vi "UI Main - SuNLaMP v1.3.0.vi"() -> ()   [LabVIEW 2017]
uses:
  e1ad3939-0f1a-413b-8e12-73ea7a7ed0d6.vi
  13f53db5-d547-40ce-b72e-27caf69f0b89.vi
  76f48c83-6457-427b-80e1-e30a4e2751fa.vi
  Globals/Global - All UI Loop Stop.vi
  support/Match 1D Array Elements/Match 1D Array Elements - string.vi
  support/Delete Elements From Array/Delete Elements From Array - double.vi
  Globals/Global - Configuration Options.vi
  Globals/Global - UI Stream and Variable Connections.vi
  support/User Event - Stop/User Event - Stop.lvlib
  support/Message Queue/Message Queue.lvlib
panel:
  in  "Temp To Monitor":string="Recup Cold Outlet Temperature [F]\nRecup Hot Inlet Temperature [F]\nPump Outlet Temperature [F]\nPump Inlet Temperature [F]\nCooler Outlet Temperature [F]\nCooler Inlet Temperature [F]\nWater Inlet Temperature [F]\nWater Outlet Temperature [F]\nRecup Hot Outlet Temperature [F]\nRecup Cold Inlet Temperature [F]\nHeater Inlet Temperature [F]"
  in  "Temp Alert Limit":dbl=140.0 format="%#_13g"
  in  "Alarm":bool
  in  "Temp Alert":bool
  out "time":timestamp format="%<%Y-%m-%d %H:%M:%S%2u>T"
  in  "clear?":bool
  in  "pump map":path=path "C:/LabView/7.5 hp Magnepump Curves.txt"
  in  "Refresh Map?":bool
  out "Map":cluster{dbl[], dbl[]}[](graph)=[{[15.211267605633802], [164.25819822966048]}, {[15.211267605633802, 15.211267605633802, 15.211267605633802, 15.211267605633802, 15.211267605633802, 15.211267605633802, 15.211267605633802, 15.211267605633802, 15.211267605633802, 15.211267605633802, 15.211267605633802, 15.211267605633802, 15.211267605633802, 15.211267605633802, 15.211267605633802, 15.211267605633802, 15.211267605633802, 15.211267605633802, 15.211267605633802, 15.211267605633802, 15.211267605633802, 15.211267605633802, 15.211267605633802, 15.211267605633802, 15.211267605633802, 15.211267605633802, 15.211267605633802, 15.211267605633802, 15.211267605633802, 15.211267605633802, 15.211267605633802, 15.211267605633802, 15.211267605633802, 15.211267605633802, 15.211267605633802, 15.211267605633802, 15.211267605633802, 15.211267605633802, 15.211267605633802, 15.211267605633802, 15.211267605633802, 15.211267605633802, 15.211267605633802, 15.211267605633802, 15.211267605633802, 15.211267605633802, 15.211267605633802, 15.211267605633802, 15.211267605633802, 15.211267605633802, 15.211267605633802, 15.211267605633802, 15.211267605633802, 15.211267605633802, 15.211267605633802, 15.211267605633802, 15.211267605633802, 15.211267605633802, 15.211267605633802, 15.211267605633802, 15.211267605633802, 15.211267605633802, 15.211267605633802, 15.211267605633802, 15.211267605633802, 15.211267605633802, 15.211267605633802, 15.211267605633802, 15.211267605633802, 15.211267605633802, 15.211267605633802, 15.211267605633802, 15.211267605633802], [164.25819822966048, 164.25819822966048, 164.25819822966048, 164.25819822966048, 164.25819822966048, 164.25819822966048, 164.25819822966048, 164.25819822966048, 164.25819822966048, 164.25819822966048, 164.25819822966048, 164.25819822966048, 164.25819822966048, 164.25819822966048, 164.25819822966048, 164.25819822966048, 164.25819822966048, 164.25819822966048, 164.25819822966048, 164.25819822966048, 164.25819822966048, 164.25819822966048, 164.25819822966048, 164.25819822966048, 164.25819822966048, 164.25819822966048, 164.25819822966048, 164.25819822966048, 164.25819822966048, 164.25819822966048, 164.25819822966048, 164.25819822966048, 164.25819822966048, 164.25819822966048, 164.25819822966048, 164.25819822966048, 164.25819822966048, 164.25819822966048, 164.25819822966048, 164.25819822966048, 164.25819822966048, 164.25819822966048, 164.25819822966048, 164.25819822966048, 164.25819822966048, 164.25819822966048, 164.25819822966048, 164.25819822966048, 164.25819822966048, 164.25819822966048, 164.25819822966048, 164.25819822966048, 164.25819822966048, 164.25819822966048, 164.25819822966048, 164.25819822966048, 164.25819822966048, 164.25819822966048, 164.25819822966048, 164.25819822966048, 164.25819822966048, 164.25819822966048, 164.25819822966048, 164.25819822966048, 164.25819822966048, 164.25819822966048, 164.25819822966048, 164.25819822966048, 164.25819822966048, 164.25819822966048, 164.25819822966048, 164.25819822966048, 164.25819822966048]}, {[0.0, 0.5050505050505051, 1.0101010101010102, 1.5151515151515151, 2.0202020202020203, 2.525252525252525, 3.0303030303030303, 3.535353535353535, 4.040404040404041, 4.545454545454546, 5.05050505050505, 5.555555555555555, 6.0606060606060606, 6.565656565656567, 7.07070707070707, 7.575757575757576, 8.080808080808081, 8.585858585858585, 9.090909090909092, 9.595959595959595, 10.1010101010101, 10.606060606060606, 11.11111111111111, 11.616161616161616, 12.121212121212121, 12.626262626262626, 13.131313131313133, 13.636363636363635, 14.14141414141414, 14.646464646464647, 15.151515151515152, 15.656565656565657, 16.161616161616163, 16.666666666666664, 17.17171717171717, 17.67676767676768, 18.181818181818183, 18.68686868686869, 19.19191919191919, 19.696969696969695, 20.2020202020202, 20.707070707070706, 21.21212121212121, 21.71717171717172, 22.22222222222222, 22.727272727272727, 23.232323232323232, 23.737373737373737, 24.242424242424242, 24.747474747474747, 25.252525252525253, 25.757575757575758, 26.262626262626267, 26.767676767676768, 27.27272727272727, 27.77777777777778, 28.28282828282828, 28.78787878787879, 29.292929292929294, 29.797979797979796, 30.303030303030305, 30.808080808080806, 31.313131313131315, 31.818181818181817, 32.323232323232325, 32.82828282828283, 33.33333333333333, 33.83838383838384, 34.34343434343434, 34.84848484848485, 35.35353535353536, 35.858585858585855, 36.36363636363637, 36.868686868686865, 37.37373737373738, 37.878787878787875, 38.38383838383838, 38.88888888888889, 39.39393939393939, 39.8989898989899, 40.4040404040404, 40.909090909090914, 41.41414141414141, 41.91919191919192, 42.42424242424242, 42.92929292929293, 43.43434343434344, 43.93939393939394, 44.44444444444444, 44.94949494949495, 45.45454545454545, 45.95959595959596, 46.464646464646464, 46.96969696969697, 47.474747474747474, 47.97979797979798, 48.484848484848484, 48.98989898989899, 49.494949494949495, 50.0], [320.0, 319.9999997193249, 319.99999455484533, 319.99996914478146, 319.9998943628826, 319.9997255914889, 319.99940140243217, 319.99884246717903, 319.99795061825614, 319.9966080194432, 319.9946764186028, 319.99199646578484, 319.9883870844086, 319.98364488659047, 319.977543625857, 319.96983368198966, 319.960241573831, 319.9484694966772, 319.9341948814863, 319.9170699735952, 319.8967214290018, 319.87274992655915, 319.8447297946612, 319.8122086511911, 319.7747070556596, 319.7317181725931, 319.68270744533976, 319.62711227955526, 319.5643417357107, 319.4937762300317, 319.41476724333677, 319.32663703729554, 319.22867837767024, 319.1201542641441, 319.0002976663747, 318.86831126594063, 318.72336720387625, 318.56460683351537, 318.3911404783842, 318.20204719490437, 317.99637453968427, 317.7731383411927, 317.5313224756226, 317.269878646766, 316.987726169734, 316.6837517583631, 316.35680931616446, 316.00571973067593, 315.62927067108876, 315.226216389027, 314.7952775223654, 314.33514090197644, 313.8444593613058, 313.32185154867767, 312.76590174224026, 312.1751596674631, 311.5481403171046, 310.8833237735713, 310.17915503359444, 309.43404383515303, 308.64636448657575, 307.8144556977579, 306.9366204134314, 306.0111256484296, 305.03620232489067, 304.0100451113468, 302.9308122636464, 301.7966254676617, 300.6055696837347, 299.35569299281417, 298.0450064442441, 296.67148390515854, 295.23306191144485, 293.72763952023706, 292.15307816390055, 290.5072015054755, 288.7877952955416, 286.99260723047416, 285.1193468120571, 283.1656852084245, 281.1292551162997, 279.0076506245035, 276.7984270787053, 274.49910094738806, 272.1071496890043, 269.6200116202959, 267.0350857857544, 264.3497318281997, 261.561269860452, 258.6669803380781, 255.6641039331887, 252.54984140926717, 249.32135349701005, 245.97576077115912, 242.51014352830754, 238.92154166566087, 235.20695456073582, 231.36334095197986, 227.38761882029425, 223.27666527144538]}, {[0.0, 0.4951475539710834, 0.9902951079421668, 1.4854426619132501, 1.9805902158843336, 2.475737769855417, 2.9708853238265003, 3.4660328777975833, 3.961180431768667, 4.456327985739751, 4.951475539710834, 5.446623093681917, 5.941770647653001, 6.436918201624085, 6.932065755595167, 7.427213309566251, 7.922360863537334, 8.417508417508417, 8.912655971479502, 9.407803525450584, 9.902951079421667, 10.39809863339275, 10.893246187363834, 11.388393741334918, 11.883541295306001, 12.378688849277085, 12.87383640324817, 13.36898395721925, 13.864131511190333, 14.359279065161418, 14.854426619132502, 15.349574173103585, 15.844721727074669, 16.339869281045747, 16.835016835016834, 17.33016438898792, 17.825311942959004, 18.320459496930088, 18.815607050901168, 19.31075460487225, 19.805902158843335, 20.301049712814418, 20.7961972667855, 21.29134482075659, 21.78649237472767, 22.281639928698752, 22.776787482669835, 23.27193503664092, 23.767082590612002, 24.262230144583086, 24.75737769855417, 25.252525252525253, 25.74767280649634, 26.24282036046742, 26.7379679144385, 27.233115468409586, 27.728263022380666, 28.223410576351753, 28.718558130322837, 29.213705684293917, 29.708853238265004, 30.204000792236084, 30.69914834620717, 31.19429590017825, 31.689443454149337, 32.18459100812042, 32.679738562091494, 33.17488611606259, 33.67003367003367, 34.165181224004755, 34.66032877797584, 35.155476331946915, 35.65062388591801, 36.14577143988908, 36.640918993860176, 37.13606654783125, 37.631214101802335, 38.12636165577342, 38.6215092097445, 39.11665676371559, 39.61180431768667, 40.106951871657756, 40.602099425628836, 41.097246979599916, 41.592394533571, 42.08754208754208, 42.58268964151318, 43.07783719548425, 43.57298474945534, 44.06813230342642, 44.563279857397504, 45.058427411368584, 45.55357496533967, 46.04872251931075, 46.54387007328184, 47.03901762725292, 47.534165181224004, 48.029312735195084, 48.52446028916617, 49.01960784313725], [307.5740099961553, 307.57400972637913, 307.5740047624426, 307.5739803390825, 307.57390846105596, 307.57374624326116, 307.5734346428606, 307.5728974117445, 307.5720401944023, 307.5707497303376, 307.56889313591194, 307.5663172489281, 307.5628480242297, 307.55828997173245, 307.5524256303892, 307.5450150730389, 307.5357954381305, 307.52448048507995, 307.51076017059427, 307.4943002437478, 307.47474185794096, 307.4517011981537, 307.4247691221272, 307.3935108142936, 307.3574654514221, 307.3161458790783, 307.26903829809663, 307.2156019603568, 307.1552688732321, 307.0874435121412, 307.01150254069273, 306.9267945379619, 306.83263973247807, 306.72832974254527, 306.6131273225439, 306.4862661148987, 306.3469504074166, 306.19435489572794, 306.02762445058073, 305.84587388975814, 305.64818775440625, 305.4336200895739, 305.20119422877985, 304.9499025824356, 304.6787064299635, 304.38653571545854, 304.0722888467555, 303.73483249776615, 303.3730014139646, 302.98559822090255, 302.5713932356453, 302.1291242810231, 301.6574965026007, 301.1551821882715, 300.6208205903885, 300.053017750349, 299.45034632555223, 298.81134541865754, 298.13452040906805, 297.41834278657535, 296.661249987097, 295.86164523044783, 295.01789736008396, 294.1283406847651, 293.19127482207864, 292.20496454377815, 291.16763962288195, 290.07749468248915, 288.9326890462656, 287.7313465905557, 286.4715555980816, 285.1513686131858, 283.7688022985821, 282.32183729357655, 280.8084180737221, 279.22645281187573, 277.57381324062055, 275.8483345160267, 274.0478150827154, 272.1700165402004, 270.21266351047643, 268.17344350682765, 266.0500068038305, 263.8399663085237, 261.5408974327223, 259.1503379664512, 256.66578795247443, 254.08470956189896, 251.40452697083043, 248.6226262380604, 245.7363551837646, 242.7430232691918, 239.63990147732605, 236.42422219450125, 233.09317909295225, 229.64392701428378, 226.07358185384064, 222.37922044596294, 218.5578804501098, 214.60656023783676]}, {[0.0, 0.4621377170396778, 0.9242754340793556, 1.3864131511190334, 1.8485508681587113, 2.3106885851983887, 2.772826302238067, 3.2349640192777445, 3.6971017363174226, 4.159239453357101, 4.621377170396777, 5.083514887436456, 5.545652604476134, 6.007790321515812, 6.469928038555489, 6.9320657555951675, 7.394203472634845, 7.856341189674522, 8.318478906714201, 8.780616623753877, 9.242754340793555, 9.704892057833234, 10.167029774872912, 10.62916749191259, 11.091305208952267, 11.553442925991945, 12.015580643031624, 12.4777183600713, 12.939856077110978, 13.401993794150657, 13.864131511190335, 14.326269228230013, 14.78840694526969, 15.250544662309366, 15.712682379349044, 16.174820096388725, 16.636957813428403, 17.09909553046808, 17.561233247507754, 18.023370964547432, 18.48550868158711, 18.947646398626787, 19.40978411566647, 19.87192183270615, 20.334059549745824, 20.7961972667855, 21.25833498382518, 21.720472700864857, 22.182610417904534, 22.644748134944212, 23.10688585198389, 23.569023569023567, 24.03116128606325, 24.493299003102923, 24.9554367201426, 25.41757443718228, 25.879712154221956, 26.341849871261637, 26.803987588301315, 27.26612530534099, 27.72826302238067, 28.190400739420344, 28.652538456460025, 29.1146761734997, 29.57681389053938, 30.038951607579058, 30.501089324618732, 30.963227041658417, 31.425364758698088, 31.887502475737772, 32.34964019277745, 32.811777909817124, 33.273915626856805, 33.73605334389648, 34.19819106093616, 34.660328777975835, 35.12246649501551, 35.5846042120552, 36.046741929094864, 36.50887964613455, 36.97101736317422, 37.43315508021391, 37.895292797253575, 38.357430514293256, 38.81956823133294, 39.28170594837261, 39.7438436654123, 40.20598138245197, 40.66811909949165, 41.13025681653132, 41.592394533571, 42.05453225061068, 42.51666996765036, 42.97880768469003, 43.440945401729714, 43.90308311876939, 44.36522083580907, 44.82735855284875, 45.289496269888424, 45.751633986928105], [267.93113759665084, 267.9311373616458, 267.93113303750556, 267.9311117620452, 267.93104914829763, 267.93090783857417, 267.930636400003, 267.9301684120085, 267.9294216804571, 267.9282975428718, 267.9266802428388, 267.92443635906625, 267.9214142788845, 267.91744370870913, 267.91233521580574, 267.9058797969583, 267.89784847054926, 267.8879918892252, 267.87603997082874, 267.8617015456647, 267.844664018473, 267.82459304372503, 267.80113221305305, 267.7739027537846, 267.74250323768325, 267.70650929910823, 267.6654733618975, 267.6189243743553, 267.5663675517933, 267.5072841261319, 267.4411311021146, 267.36734101973565, 267.28532172251425, 267.19445613128386, 267.0941020231938, 266.98359181564507, 266.86223235490513, 266.7293047091674, 266.5840639658392, 266.425739032856, 266.2535324438383, 266.0666201669177, 265.86415141707045, 265.64524847181053, 265.4090064901015, 265.154493334355, 264.8807493953959, 264.58678742027627, 264.27159234283135, 263.9341211168751, 263.5733025519399, 263.18803715146896, 262.7771969533766, 262.33962537289426, 261.87413704762736, 261.3795176847484, 260.8545239102588, 260.2978831202528, 259.7082933341215, 259.084423049639, 258.42491109987117, 257.72836651185673, 256.9933683670065, 256.2184656631731, 255.40217717834406, 254.5429913359134, 253.63936607148824, 252.68972870119052, 251.69247579141353, 250.64597302999516, 249.54855509877328, 248.3985255474863, 247.19415666898706, 245.93368937573777, 244.61533307755352, 243.23726556056727, 241.79763286738498, 240.29454917840545, 238.72609669427646, 237.09032551946345, 235.3852535469039, 233.60886634372542, 231.75911703800347, 229.83392620653618, 227.83118176361586, 225.74873885077528, 223.5844197274888, 221.33601366280976, 219.0012768279234, 216.5779321895993, 214.0636694045238, 211.45614471449596, 208.7529808424707, 205.95176688943218, 203.05005823208285, 200.04537642133164, 196.93520908156785, 193.7170098107055, 190.38819808098452, 186.94615914051556]}, {[0.0, 0.4291278801082723, 0.8582557602165446, 1.2873836403248167, 1.7165115204330892, 2.145639400541361, 2.5747672806496333, 3.0038951607579056, 3.4330230408661784, 3.8621509209744507, 4.291278801082722, 4.720406681190995, 5.149534561299267, 5.57866244140754, 6.007790321515811, 6.436918201624084, 6.866046081732357, 7.295173961840628, 7.724301841948901, 8.153429722057172, 8.582557602165444, 9.011685482273716, 9.44081336238199, 9.869941242490262, 10.299069122598533, 10.728197002706807, 11.15732488281508, 11.586452762923349, 12.015580643031623, 12.444708523139896, 12.873836403248168, 13.30296428335644, 13.732092163464714, 14.161220043572982, 14.590347923681255, 15.01947580378953, 15.448603683897803, 15.877731564006075, 16.306859444114345, 16.735987324222616, 17.16511520433089, 17.59424308443916, 18.023370964547432, 18.452498844655707, 18.88162672476398, 19.31075460487225, 19.739882484980523, 20.169010365088795, 20.598138245197067, 21.027266125305342, 21.456394005413614, 21.885521885521886, 22.31464976563016, 22.74377764573843, 23.172905525846698, 23.602033405954973, 24.031161286063245, 24.46028916617152, 24.889417046279792, 25.31854492638806, 25.747672806496336, 26.176800686604604, 26.60592856671288, 27.03505644682115, 27.464184326929427, 27.8933122070377, 28.322440087145964, 28.751567967254243, 29.18069584736251, 29.609823727470786, 30.03895160757906, 30.468079487687326, 30.897207367795605, 31.32633524790387, 31.75546312801215, 32.184591008120414, 32.61371888822869, 33.042846768336965, 33.47197464844523, 33.90110252855351, 34.33023040866178, 34.75935828877006, 35.18848616887832, 35.617614048986596, 36.046741929094864, 36.47586980920314, 36.904997689311415, 37.33412556941968, 37.76325344952796, 38.19238132963623, 38.6215092097445, 39.05063708985278, 39.479764969961046, 39.90889285006932, 40.33802073017759, 40.767148610285865, 41.19627649039413, 41.62540437050241, 42.054532250610684, 42.48366013071895], [231.02225639711222, 231.02225619448035, 231.02225246601247, 231.02223412135532, 231.02218013297093, 231.02205828938284, 231.02182424285974, 231.02142072259923, 231.02077685712882, 231.01980757523134, 231.01841306652943, 231.0164782891949, 231.01387251597697, 231.01044891210128, 231.00604414015905, 231.00047798819364, 230.9935530179736, 230.98505423101562, 230.97474875035746, 230.96238551641497, 230.9476949955201, 230.9303888999466, 230.9101599183978, 230.88668145606943, 230.8596073835126, 230.82857179361883, 230.79318876612592, 230.75305213911247, 230.70773528700545, 230.65679090467495, 230.59975079723145, 230.53612567518024, 230.4654049546169, 230.38705656217846, 230.30052674448854, 230.20523988185727, 230.10059830601514, 229.9859821216801, 229.86074903176953, 229.72423416608498, 229.57574991330958, 229.41458575616883, 229.24000810961687, 229.0512601619183, 228.8475617185059, 228.6281090485, 228.39207473378525, 228.13860752054438, 227.86683217315561, 227.5758493303668, 227.26473536366248, 226.93254223774625, 226.57829737306452, 226.2010035103017, 225.79963857678072, 225.37315555470659, 224.9204823511926, 224.44052167001388, 223.93215088503337, 223.39422191524994, 222.82556110141954, 222.22496908420302, 221.59122068379642, 220.92306478100133, 220.21922419969465, 219.47839559066006, 218.69924931674242, 217.88042933929185, 217.0205531058617, 216.11821143912852, 215.17196842700352, 214.18036131390403, 213.14190039315724, 212.05506890050862, 210.91832290870687, 209.7300912231422, 208.48877527851056, 207.19274903648227, 205.84035888435065, 204.4299235346394, 202.95973392564676, 201.42805312290614, 199.8331162215438, 198.17313024951335, 196.4462740716892, 194.65069829480115, 192.7845251731919, 190.8458485153819, 188.83273359142376, 186.74321704103207, 184.57530678247207, 182.32698192219297, 179.9961926651916, 177.58086022609206, 175.0788767409286, 172.4881051796176, 169.806379259107, 167.03150335718996, 164.16125242697137, 161.19337191197516]}, {[0.0, 0.3961180431768667, 0.7922360863537334, 1.1883541295306002, 1.5844721727074669, 1.9805902158843334, 2.3767082590612003, 2.772826302238067, 3.1689443454149337, 3.5650623885918007, 3.9611804317686667, 4.357298474945534, 4.753416518122401, 5.149534561299268, 5.545652604476134, 5.941770647653001, 6.3378886908298675, 6.734006734006733, 7.130124777183601, 7.5262428203604665, 7.9223608635373335, 8.3184789067142, 8.714596949891067, 9.110714993067933, 9.506833036244801, 9.902951079421667, 10.299069122598535, 10.6951871657754, 11.091305208952267, 11.487423252129135, 11.883541295306001, 12.279659338482869, 12.675777381659735, 13.0718954248366, 13.468013468013465, 13.864131511190335, 14.260249554367203, 14.656367597544069, 15.052485640720933, 15.448603683897801, 15.844721727074667, 16.240839770251533, 16.6369578134284, 17.03307585660527, 17.429193899782135, 17.825311942959, 18.221429986135867, 18.617548029312733, 19.013666072489602, 19.40978411566647, 19.805902158843335, 20.2020202020202, 20.59813824519707, 20.994256288373936, 21.3903743315508, 21.78649237472767, 22.182610417904534, 22.578728461081404, 22.97484650425827, 23.370964547435133, 23.767082590612002, 24.16320063378887, 24.559318676965738, 24.9554367201426, 25.35155476331947, 25.747672806496336, 26.1437908496732, 26.53990889285007, 26.93602693602693, 27.332144979203804, 27.72826302238067, 28.124381065557532, 28.520499108734406, 28.916617151911264, 29.312735195088138, 29.708853238265, 30.104971281441866, 30.50108932461874, 30.897207367795602, 31.29332541097247, 31.689443454149334, 32.0855614973262, 32.481679540503066, 32.877797583679936, 33.2739156268568, 33.67003367003367, 34.06615171321054, 34.4622697563874, 34.85838779956427, 35.25450584274113, 35.650623885918, 36.04674192909487, 36.442859972271734, 36.8389780154486, 37.235096058625466, 37.631214101802335, 38.027332144979205, 38.42345018815607, 38.81956823133294, 39.21568627450981], [196.8473663975394, 196.84736622488265, 196.84736304796328, 196.8473474170128, 196.8473014150758, 196.84719759568713, 196.84699817143078, 196.8466543435165, 196.84610572441744, 196.84527982741605, 196.84409160698365, 196.842443039314, 196.840222735507, 196.83730558190877, 196.83355240344912, 196.82880964674487, 196.82290908040352, 196.81566751045116, 196.80688650918032, 196.79635215599856, 196.78383478908222, 196.76908876681838, 196.75185223816143, 196.7318469211479, 196.70877788891013, 196.68233336261014, 196.65218451078184, 196.61798525462837, 196.57937207886854, 196.53596384777035, 196.48736162604337, 196.4331485042956, 196.37288942878598, 196.30613103522896, 196.2324014864281, 196.15121031353516, 196.06204826074662, 195.9643871332659, 195.85767964837166, 195.7413592894452, 195.61484016282, 195.4775168573273, 195.32876430641912, 195.16793765275878, 194.99437211517662, 194.80738285789346, 194.60626486192353, 194.39029279857036, 194.15872090493733, 193.9107828613776, 193.645691670813, 193.36263953985477, 193.06079776166445, 192.73931660049374, 192.39732517784867, 192.03393136022336, 191.64822164835346, 191.23926106794082, 190.80609306180358, 190.34773938340822, 189.86319999174208, 189.3514529474866, 188.81145431045374, 188.24213803824964, 187.64241588613035, 187.01117730801803, 186.34728935864445, 185.64959659679306, 184.91692098960996, 184.14806181795564, 183.34179558277222, 182.49687591243892, 181.61203347109256, 180.685975867889, 179.7173875671822, 178.70492979960045, 177.64724047399716, 176.54293409025706, 175.39060165293782, 174.18881058572825, 172.93610464670493, 171.6310038443697, 170.27200435445152, 168.85757843745515, 167.38617435694226, 165.85621629852878, 164.26610428958364, 162.61421411961535, 160.89889726133148, 159.11848079235867, 157.27126731760933, 155.35553489228275, 153.36953694548868, 151.3115022044808, 149.17963461948943, 146.97211328914162, 144.687092386458, 142.3227010854163, 139.87704348807029, 137.34819855221554]}, {[0.0, 0.3631082062454612, 0.7262164124909224, 1.0893246187363834, 1.4524328249818448, 1.8155410312273057, 2.178649237472767, 2.541757443718228, 2.9048656499636896, 3.2679738562091507, 3.6310820624546114, 3.9941902687000725, 4.357298474945534, 4.720406681190996, 5.083514887436456, 5.446623093681917, 5.809731299927379, 6.1728395061728385, 6.535947712418301, 6.899055918663761, 7.262164124909223, 7.625272331154684, 7.988380537400145, 8.351488743645605, 8.714596949891067, 9.07770515613653, 9.440813362381991, 9.80392156862745, 10.167029774872912, 10.530137981118374, 10.893246187363834, 11.256354393609296, 11.619462599854758, 11.982570806100217, 12.345679012345677, 12.70878721859114, 13.071895424836603, 13.435003631082063, 13.798111837327522, 14.161220043572984, 14.524328249818446, 14.887436456063906, 15.250544662309368, 15.613652868554832, 15.97676107480029, 16.33986928104575, 16.70297748729121, 17.066085693536674, 17.429193899782135, 17.792302106027595, 18.15541031227306, 18.51851851851852, 18.881626724763983, 19.24473493100944, 19.6078431372549, 19.970951343500364, 20.334059549745824, 20.697167755991288, 21.060275962236748, 21.423384168482205, 21.78649237472767, 22.14960058097313, 22.512708787218592, 22.875816993464053, 23.238925199709517, 23.602033405954977, 23.965141612200433, 24.328249818445897, 24.691358024691354, 25.05446623093682, 25.41757443718228, 25.78068264342774, 26.143790849673206, 26.506899055918662, 26.870007262164126, 27.233115468409583, 27.596223674655043, 27.95933188090051, 28.322440087145967, 28.685548293391435, 29.04865649963689, 29.411764705882355, 29.77487291212781, 30.137981118373272, 30.501089324618736, 30.864197530864196, 31.227305737109663, 31.59041394335512, 31.95352214960058, 32.316630355846044, 32.6797385620915, 33.042846768336965, 33.40595497458242, 33.769063180827885, 34.13217138707335, 34.495279593318806, 34.85838779956427, 35.22149600580973, 35.58460421205519, 35.947712418300654], [165.40646759793242, 165.40646745285278, 165.40646478335802, 165.4064516490177, 165.4064129946123, 165.4063257574871, 165.40615818571612, 165.4058692747604, 165.40540828232298, 165.40471429942596, 165.40371586420153, 165.40233060942356, 165.40046493747462, 165.39801371813166, 165.39486000567598, 165.390874772612, 165.3859166578391, 165.3798317275319, 165.37245324729736, 165.36360146441544, 165.35308339915935, 165.34069264434044, 165.32620917234397, 165.30939914902012, 165.29001475387588, 165.2677940060821, 165.2424605958653, 165.213723720903, 165.18127792738258, 165.14480295541813, 165.10396358855033, 165.0584095070817, 165.00777514502155, 164.95167955043544, 164.8897262490125, 164.82150311067886, 164.7465822190996, 164.6645197439248, 164.57485581564563, 164.4771144029366, 164.37080319236958, 164.25541347039305, 164.13042000747717, 163.99528094433202, 163.84943768011368, 163.6923147625355, 163.52331977981075, 163.34184325435425, 163.1472585381765, 162.93892170990756, 162.71617147339146, 162.47832905779464, 162.22469811917637, 161.95456464347043, 161.66719685083117, 161.3618451012988, 161.03774180174142, 160.6941013140336, 160.33011986443216, 159.94497545411386, 159.53782777083885, 159.1078181017075, 158.6540692469785, 158.17568543491808, 157.6717522376512, 157.14133648798736, 156.58348619719428, 155.99723047369417, 155.38157944265836, 154.7355241664766, 154.05803656607944, 153.34806934309103, 152.60455590279304, 151.82641027787895, 151.01252705297946, 150.16178128994204, 149.27302845384483, 148.3451043397299, 147.37682500003802, 146.36698667272998, 145.31436571007845, 144.2177185081162, 143.07578143672663, 141.88727077036162, 140.6508826193751, 139.3652928619582, 138.029157076664, 136.64111047551012, 135.1997678376466, 133.70372344357915, 132.15155100993562, 130.54180362476538, 128.87301368336202, 127.14369282459845, 125.35233186776543, 123.49740074990372, 121.57734846362096, 119.59060299538451, 117.53557126428127, 115.41063906123665]}, {[0.0, 0.3300983693140556, 0.6601967386281112, 0.9902951079421668, 1.3203934772562225, 1.6504918465702778, 1.9805902158843336, 2.310688585198389, 2.640786954512445, 2.9708853238265007, 3.3009836931405556, 3.6310820624546114, 3.961180431768667, 4.291278801082723, 4.621377170396778, 4.9514755397108345, 5.28157390902489, 5.611672278338944, 5.9417706476530014, 6.271869016967056, 6.601967386281111, 6.9320657555951675, 7.262164124909223, 7.592262494223278, 7.922360863537334, 8.25245923285139, 8.582557602165446, 8.9126559714795, 9.242754340793557, 9.572852710107613, 9.902951079421669, 10.233049448735724, 10.56314781804978, 10.893246187363832, 11.223344556677889, 11.553442925991947, 11.883541295306003, 12.213639664620057, 12.543738033934112, 12.873836403248168, 13.203934772562222, 13.534033141876279, 13.864131511190335, 14.194229880504393, 14.524328249818446, 14.854426619132502, 15.184524988446556, 15.514623357760613, 15.844721727074669, 16.174820096388725, 16.50491846570278, 16.835016835016834, 17.165115204330892, 17.495213573644946, 17.825311942959, 18.15541031227306, 18.485508681587113, 18.81560705090117, 19.145705420215226, 19.47580378952928, 19.805902158843338, 20.13600052815739, 20.466098897471447, 20.7961972667855, 21.12629563609956, 21.456394005413614, 21.786492374727665, 22.116590744041726, 22.446689113355777, 22.77678748266984, 23.106885851983893, 23.436984221297944, 23.767082590612006, 24.097180959926057, 24.427279329240115, 24.757377698554166, 25.087476067868224, 25.41757443718228, 25.747672806496336, 26.077771175810394, 26.407869545124445, 26.737967914438507, 27.068066283752557, 27.398164653066612, 27.72826302238067, 28.058361391694724, 28.388459761008786, 28.718558130322837, 29.04865649963689, 29.378754868950946, 29.708853238265004, 30.038951607579058, 30.369049976893113, 30.69914834620717, 31.029246715521225, 31.35934508483528, 31.689443454149337, 32.01954182346339, 32.34964019277745, 32.6797385620915], [136.69955999829125, 136.69955987839074, 136.69955767219673, 136.69954681737002, 136.69951487158045, 136.69944277478274, 136.69930428571584, 136.6990655163309, 136.69868453084547, 136.69811099126116, 136.6972858381831, 136.69614099952364, 136.6945991218799, 136.69257332076998, 136.68996694683966, 136.68667336579506, 136.68257575028025, 136.67754688225776, 136.6714489647086, 136.66413344166568, 136.65544082575155, 136.64520053251277, 136.63323072094545, 136.61933813968608, 136.60331797840985, 136.58495372403482, 136.5640170213763, 136.5402675379364, 136.5134528325476, 136.48330822761832, 136.44955668475234, 136.41190868353863, 136.37006210332362, 136.3237021077979, 136.27250103224176, 136.21611827328832, 136.15420018107406, 136.0863799536569, 136.01227753359146, 135.93149950655916, 135.84363900195834, 135.74827559536618, 135.64497521279105, 135.53329003663805, 135.4127584133171, 135.28290476242603, 135.14323948744692, 134.99325888789608, 134.83244507287316, 134.6602658759567, 134.47617477139792, 134.27961079156583, 134.06999844560033, 133.84674763923178, 133.60925359572826, 133.3568967779329, 133.08904281135656, 132.80504240829225, 132.50423129291914, 132.18593012736684, 131.84944443870978, 131.4940645468657, 131.11906549337067, 130.7237069710067, 130.3072332542572, 129.8688731305681, 129.40783983239197, 128.9233309699952, 128.41452846500692, 127.88059848469143, 127.32069137692517, 126.73394160586038, 126.11946768825872, 125.47637213047848, 124.80374136609875, 124.100645694167, 123.36613921805359, 122.59925978490075, 121.79902892565129, 120.96445179564464, 120.09451711576732, 119.18819711414564, 118.24444746836913, 117.26220724823276, 116.2403988589877, 115.17792798508945, 114.07368353443309, 112.92653758306622, 111.73534532036909, 110.49894499469353, 109.21615785945095, 107.88578811964081, 106.5066228788116, 105.07743208644501, 103.59696848575656, 102.06396756190392, 100.47714749059585, 98.83520908709465, 97.13683575560437, 95.38069343903857]}, {[0.0, 0.29708853238265004, 0.5941770647653001, 0.8912655971479501, 1.1883541295306002, 1.4854426619132501, 1.7825311942959001, 2.07961972667855, 2.3767082590612003, 2.6737967914438507, 2.9708853238265003, 3.2679738562091503, 3.5650623885918002, 3.862150920974451, 4.1592394533571, 4.456327985739751, 4.753416518122401, 5.05050505050505, 5.3475935828877015, 5.64468211527035, 5.941770647653001, 6.23885918003565, 6.5359477124183005, 6.833036244800951, 7.1301247771836005, 7.427213309566251, 7.724301841948902, 8.02139037433155, 8.3184789067142, 8.615567439096852, 8.912655971479502, 9.209744503862153, 9.506833036244801, 9.80392156862745, 10.1010101010101, 10.398098633392753, 10.695187165775403, 10.992275698158053, 11.2893642305407, 11.58645276292335, 11.883541295306001, 12.180629827688652, 12.4777183600713, 12.774806892453952, 13.071895424836601, 13.368983957219251, 13.666072489601902, 13.963161021984552, 14.260249554367201, 14.557338086749851, 14.854426619132502, 15.151515151515152, 15.448603683897804, 15.745692216280453, 16.0427807486631, 16.339869281045754, 16.6369578134284, 16.93404634581105, 17.231134878193703, 17.528223410576352, 17.825311942959004, 18.122400475341653, 18.419489007724305, 18.71657754010695, 19.013666072489602, 19.310754604872255, 19.6078431372549, 19.904931669637556, 20.2020202020202, 20.499108734402853, 20.796197266785505, 21.09328579916815, 21.390374331550806, 21.68746286393345, 21.984551396316107, 22.281639928698752, 22.5787284610814, 22.875816993464056, 23.1729055258467, 23.469994058229357, 23.767082590612002, 24.064171122994654, 24.361259655377303, 24.65834818775995, 24.9554367201426, 25.252525252525253, 25.549613784907905, 25.846702317290553, 26.143790849673202, 26.440879382055854, 26.737967914438503, 27.03505644682115, 27.332144979203804, 27.629233511586452, 27.926322043969105, 28.223410576351753, 28.520499108734402, 28.817587641117054, 29.114676173499703, 29.411764705882355], [110.72664359861592, 110.72664350149651, 110.72664171447936, 110.72663292206971, 110.72660704598016, 110.72654864757403, 110.72643647142982, 110.72624306822804, 110.72593446998484, 110.72546990292153, 110.72480152892831, 110.72387420961414, 110.72262528872271, 110.7209843898237, 110.71887322694015, 110.71620542629401, 110.712886357727, 110.7088129746288, 110.70387366141395, 110.69794808774921, 110.69090706885876, 110.68261243133536, 110.67291688396583, 110.66166389314571, 110.64868756251197, 110.63381251646821, 110.61685378731481, 110.59761670572847, 110.57589679436357, 110.55147966437085, 110.52414091464941, 110.49364603366628, 110.45975030369213, 110.42219870731631, 110.38072583611583, 110.33505580136355, 110.28490214666999, 110.22996776246208, 110.16994480220907, 110.10451460031294, 110.03334759158626, 109.95610323224662, 109.87242992236077, 109.78196492967683, 109.68433431478687, 109.57915285756509, 109.466023984832, 109.34453969919583, 109.21428050902726, 109.07481535952492, 108.92570156483232, 108.76648474116833, 108.59669874093626, 108.41586558777774, 108.22349541253989, 108.01908639012565, 107.80212467719883, 107.57208435071672, 107.32842734726452, 107.07060340316715, 106.79804999535494, 106.51019228296123, 106.20644304963025, 105.88620264651543, 105.54885893594833, 105.19378723576015, 104.8203502642375, 104.42789808569611, 104.01576805665562, 103.58328477260007, 103.12976001530939, 102.65449270074691, 102.15676882748957, 101.63586142568758, 101.09103050654, 100.52152301227527, 99.92657276662341, 99.30540042576962, 98.65721342977754, 97.98120595447216, 97.27655886377153, 96.54243966245798, 95.778002449379, 94.98238787106854, 94.15472307578004, 93.29412166792245, 92.39968366289081, 91.47049544228365, 90.50562970949898, 89.50414544570177, 88.46508786615527, 87.38748837690906, 86.2703645318374, 85.11271999002047, 83.91354447346282, 82.67181372514217, 81.38648946738265, 80.05651936054667, 78.68083696203954, 77.25836168562124]}, {[0.0, 0.2640786954512445, 0.528157390902489, 0.7922360863537334, 1.056314781804978, 1.3203934772562222, 1.5844721727074669, 1.8485508681587113, 2.112629563609956, 2.3767082590612008, 2.6407869545124445, 2.904865649963689, 3.1689443454149337, 3.433023040866179, 3.6971017363174226, 3.9611804317686676, 4.225259127219912, 4.489337822671156, 4.7534165181224015, 5.017495213573644, 5.281573909024889, 5.545652604476134, 5.809731299927378, 6.073809995378623, 6.3378886908298675, 6.601967386281112, 6.866046081732358, 7.1301247771836005, 7.394203472634845, 7.658282168086091, 7.922360863537335, 8.18643955898858, 8.450518254439825, 8.714596949891067, 8.978675645342312, 9.242754340793558, 9.506833036244803, 9.770911731696048, 10.034990427147289, 10.299069122598533, 10.563147818049778, 10.827226513501023, 11.091305208952267, 11.355383904403514, 11.619462599854756, 11.883541295306001, 12.147619990757246, 12.41169868620849, 12.675777381659735, 12.93985607711098, 13.203934772562224, 13.468013468013469, 13.732092163464715, 13.996170858915958, 14.260249554367201, 14.524328249818447, 14.78840694526969, 15.052485640720937, 15.316564336172181, 15.580643031623424, 15.84472172707467, 16.108800422525913, 16.37287911797716, 16.636957813428403, 16.90103650887965, 17.165115204330892, 17.429193899782135, 17.69327259523338, 17.957351290684624, 18.22142998613587, 18.485508681587117, 18.749587377038356, 19.013666072489606, 19.277744767940845, 19.541823463392095, 19.805902158843335, 20.069980854294577, 20.334059549745827, 20.598138245197067, 20.862216940648317, 21.126295636099556, 21.390374331550806, 21.654453027002045, 21.91853172245329, 22.182610417904534, 22.44668911335578, 22.710767808807027, 22.97484650425827, 23.238925199709513, 23.50300389516076, 23.767082590612002, 24.03116128606325, 24.29523998151449, 24.559318676965738, 24.82339737241698, 25.087476067868227, 25.35155476331947, 25.615633458770716, 25.87971215422196, 26.143790849673206], [87.48771839890642, 87.48771832217008, 87.48771691020592, 87.48770996311683, 87.48768951781149, 87.48764337586097, 87.48755474285814, 87.4874019304518, 87.48715809974111, 87.48679103440715, 87.4862629364372, 87.48553023969514, 87.48454343800314, 87.4832469252928, 87.48157884597741, 87.47947095410885, 87.47684848017937, 87.47363000464499, 87.4697273374135, 87.46504540266605, 87.459482128481, 87.45292834080819, 87.4452676614051, 87.4363764093991, 87.42612350618231, 87.4143703833823, 87.40097089368085, 87.3857712242793, 87.36860981283048, 87.34931726567574, 87.32771627824152, 87.30362155746472, 87.27683974612712, 87.24716934899067, 87.21440066063474, 87.17831569490454, 87.1386881158874, 87.09528317034041, 87.04785762149854, 86.99615968419789, 86.93992896125336, 86.87889638103437, 86.8127841361863, 86.74130562344837, 86.66416538452296, 86.58105904795268, 86.49167327196604, 86.39568568825351, 86.29276484663883, 86.1825701606123, 86.06475185369469, 85.93895090660214, 85.80479900518422, 85.66191848910836, 85.5099223012661, 85.34841393787707, 85.17698739926821, 84.99522714130705, 84.80270802746827, 84.59899528151479, 84.38364444077428, 84.15620130999406, 83.91620191575724, 83.6631724614443, 83.39662928272462, 83.11607880356358, 82.82101749273087, 82.51093182079693, 82.18529821760444, 81.84358303020254, 81.48524248123212, 81.10972262775066, 80.7164593204856, 80.30487816350625, 79.87439447430322, 79.42441324426689, 78.9543290995543, 78.4635262623365, 77.95137851241684, 77.41724914921258, 76.86049095409109, 76.28044615305322, 75.67644637975626, 75.04781263886898, 74.39385526975214, 73.71387391045725, 73.00715746203718, 72.27298405316239, 71.51062100503623, 70.71932479660387, 69.89834103004861, 69.04690439657013, 68.16423864243943, 67.24955653532481, 66.30205983088422, 65.32093923961851, 64.30537439398135, 63.25453381574059, 62.1675748835868, 61.0436438009847]}, {[0.0, 0.2310688585198389, 0.4621377170396778, 0.6932065755595167, 0.9242754340793556, 1.1553442925991944, 1.3864131511190334, 1.6174820096388722, 1.8485508681587113, 2.0796197266785503, 2.3106885851983887, 2.541757443718228, 2.772826302238067, 3.003895160757906, 3.2349640192777445, 3.4660328777975837, 3.6971017363174226, 3.928170594837261, 4.159239453357101, 4.390308311876939, 4.621377170396777, 4.852446028916617, 5.083514887436456, 5.314583745956295, 5.545652604476134, 5.7767214629959724, 6.007790321515812, 6.23885918003565, 6.469928038555489, 6.700996897075329, 6.9320657555951675, 7.163134614115006, 7.394203472634845, 7.625272331154683, 7.856341189674522, 8.087410048194362, 8.318478906714201, 8.54954776523404, 8.780616623753877, 9.011685482273716, 9.242754340793555, 9.473823199313394, 9.704892057833234, 9.935960916353075, 10.167029774872912, 10.39809863339275, 10.62916749191259, 10.860236350432428, 11.091305208952267, 11.322374067472106, 11.553442925991945, 11.784511784511784, 12.015580643031624, 12.246649501551461, 12.4777183600713, 12.70878721859114, 12.939856077110978, 13.170924935630818, 13.401993794150657, 13.633062652670494, 13.864131511190335, 14.095200369710172, 14.326269228230013, 14.55733808674985, 14.78840694526969, 15.019475803789529, 15.250544662309366, 15.481613520829208, 15.712682379349044, 15.943751237868886, 16.174820096388725, 16.405888954908562, 16.636957813428403, 16.86802667194824, 17.09909553046808, 17.330164388987917, 17.561233247507754, 17.7923021060276, 18.023370964547432, 18.254439823067276, 18.48550868158711, 18.716577540106954, 18.947646398626787, 19.178715257146628, 19.40978411566647, 19.640852974186306, 19.87192183270615, 20.102990691225983, 20.334059549745824, 20.56512840826566, 20.7961972667855, 21.02726612530534, 21.25833498382518, 21.489403842345016, 21.720472700864857, 21.951541559384694, 22.182610417904534, 22.413679276424375, 22.644748134944212, 22.875816993464053], [66.98278439916271, 66.98278434041146, 66.98278325937639, 66.9827779405113, 66.98276228707441, 66.98272695964354, 66.98265910000075, 66.98254210300213, 66.98235542011427, 66.98207438571795, 66.9816700607097, 66.98110908976656, 66.98035356972113, 66.97936092717728, 66.97808380395144, 66.97646994923957, 66.97446211763732, 66.9719979723063, 66.96900999270719, 66.96542538641617, 66.96116600461825, 66.95614826093126, 66.95028305326326, 66.94347568844616, 66.93562580942081, 66.92662732477706, 66.91636834047438, 66.90473109358882, 66.89159188794832, 66.87682103153297, 66.86028277552865, 66.84183525493391, 66.82133043062856, 66.79861403282096, 66.77352550579845, 66.74589795391127, 66.71555808872628, 66.68232617729186, 66.6460159914598, 66.606434758214, 66.56338311095958, 66.51665504172942, 66.46603785426761, 66.41131211795263, 66.35225162252537, 66.28862333358875, 66.22018734884898, 66.14669685506907, 66.06789808570784, 65.98353027921877, 65.89332563798497, 65.79700928786724, 65.69429923834414, 65.58490634322357, 65.46853426190684, 65.3448794211871, 65.2136309775647, 65.0744707800632, 64.92707333353037, 64.77110576240975, 64.60622777496779, 64.43209162796418, 64.24834209175162, 64.05461641579328, 63.850544294586015, 63.63574783397835, 63.40984151787206, 63.17243217529763, 62.92311894785338, 62.66149325749879, 62.38713877469332, 62.09963138687157, 61.798539167246766, 61.48342234393444, 61.15383326938838, 60.80931639014182, 60.449408216846244, 60.07363729460136, 59.681524173569116, 59.27258137986586, 58.846313386725974, 58.402216585931356, 57.93977925950087, 57.458481551634044, 56.957795440903965, 56.43718471269382, 55.8961049318722, 55.33400341570244, 54.75031920698085, 54.144483047399824, 53.51591735113095, 52.86403617862399, 52.18824521061767, 51.487941722358045, 50.76251455802071, 50.01134410533291, 49.23380227039196, 48.42925245267637, 47.59704952024613, 46.73653978512889]}, {[0.0, 0.19805902158843336, 0.3961180431768667, 0.5941770647653001, 0.7922360863537334, 0.9902951079421667, 1.1883541295306002, 1.3864131511190334, 1.5844721727074669, 1.7825311942959003, 1.9805902158843334, 2.178649237472767, 2.3767082590612003, 2.574767280649634, 2.772826302238067, 2.9708853238265003, 3.1689443454149337, 3.3670033670033663, 3.5650623885918007, 3.7631214101802333, 3.9611804317686667, 4.1592394533571, 4.357298474945534, 4.555357496533967, 4.753416518122401, 4.951475539710834, 5.149534561299268, 5.3475935828877, 5.545652604476134, 5.7437116260645675, 5.941770647653001, 6.1398296692414345, 6.3378886908298675, 6.5359477124183, 6.734006734006733, 6.9320657555951675, 7.130124777183601, 7.328183798772034, 7.5262428203604665, 7.7243018419489005, 7.9223608635373335, 8.120419885125767, 8.3184789067142, 8.516537928302634, 8.714596949891067, 8.9126559714795, 9.110714993067933, 9.308774014656366, 9.506833036244801, 9.704892057833234, 9.902951079421667, 10.1010101010101, 10.299069122598535, 10.497128144186968, 10.6951871657754, 10.893246187363834, 11.091305208952267, 11.289364230540702, 11.487423252129135, 11.685482273717566, 11.883541295306001, 12.081600316894434, 12.279659338482869, 12.4777183600713, 12.675777381659735, 12.873836403248168, 13.0718954248366, 13.269954446425036, 13.468013468013465, 13.666072489601902, 13.864131511190335, 14.062190532778766, 14.260249554367203, 14.458308575955632, 14.656367597544069, 14.8544266191325, 15.052485640720933, 15.25054466230937, 15.448603683897801, 15.646662705486236, 15.844721727074667, 16.0427807486631, 16.240839770251533, 16.438898791839968, 16.6369578134284, 16.835016835016834, 17.03307585660527, 17.2311348781937, 17.429193899782135, 17.627252921370566, 17.825311942959, 18.023370964547436, 18.221429986135867, 18.4194890077243, 18.617548029312733, 18.815607050901168, 19.013666072489602, 19.211725094078034, 19.40978411566647, 19.607843137254903], [49.21184159938485, 49.21184155622066, 49.21184076199082, 49.2118368542532, 49.21182535376895, 49.211799398921784, 49.211749542857696, 49.21166358587912, 49.21152643110436, 49.21131995685401, 49.21102290174591, 49.2106107598285, 49.21005568387675, 49.20932639547719, 49.20838810086228, 49.20720241168622, 49.20572727010088, 49.20391687761279, 49.20172162729508, 49.19908803899964, 49.195958697270555, 49.192272191704596, 49.18796305954036, 49.182961730286976, 49.177194472227534, 49.170583340652534, 49.16304612769546, 49.15449631365709, 49.144843019717136, 49.13399096194259, 49.12184040651084, 49.1082871260739, 49.093222357196495, 49.07653275880724, 49.058100371607026, 49.03780257838379, 49.015512065186655, 48.99109678331647, 48.964419912092914, 48.9353398223613, 48.903710040705, 48.86937921433182, 48.83219107660478, 48.791984413189695, 48.748593028794154, 48.701845714473365, 48.651566215480884, 48.59757319964259, 48.53968022623433, 48.4776957153444, 48.41142291770325, 48.34065988496369, 48.26519944041611, 48.184829150123434, 48.09933129446217, 48.00848284005584, 47.912055412088364, 47.809815266985204, 47.701523265450895, 47.586934845852056, 47.46579999793552, 47.33786323687165, 47.202863577613435, 47.06053450956241, 46.91060397153259, 46.75279432700451, 46.58682233966111, 46.412399149198265, 46.22923024740249, 46.03701545448891, 45.835448895693055, 45.62421897810973, 45.40300836777314, 45.17149396697225, 44.92934689179555, 44.67623244990011, 44.41181011849929, 44.135733522564266, 43.847650413234454, 43.54720264643206, 43.23402616167623, 42.907750961092425, 42.56800108861288, 42.21439460936379, 41.846543589235566, 41.464054074632195, 41.06652607239591, 40.65355352990384, 40.22472431533287, 39.77962019808967, 39.31781682940233, 38.83888372307069, 38.34238423637217, 37.8278755511202, 37.29490865487236, 36.743028322285404, 36.1717730966145, 35.580675271354075, 34.96926087201757, 34.337049638053884]}]
  in  "Pump Enable":bool
  out "Dead Head [psig]":dbl format="%#.1f psig"
  in  "Drive Air Pressure Cmd [psig]":dbl caption="Drive Air [psig]" min=0.0 max=148.0 step=1.0 format="%#_g psig"
  out "Water Valve % Closed":dbl format="%#.1f %%"
  in  "Water Valve % Closed Cmd":dbl caption="Water Valve % Closed" min=0.0 max=100.0 step=1.0
  out "Regulated Pressure [psig]":dbl format="%#.1f psig"
  in  "Regulated CO2 Pressure Cmd [psig]":dbl caption="Regulated CO2 Pressure [psig]" min=0.0 max=100.0 step=1.0
  out "Heater Power [%]":dbl format="%#.1f %%"
  in  "Heater Power Cmd [%]":dbl caption="Heater Power [%]" min=-1.0 max=76.5 step=1.0
  out "Cooling Valve % Closed":dbl format="%#.1f %%"
  in  "Cooling Valve % Closed Cmd":dbl caption="Cooling Valve % Closed" min=0.0 max=100.0 step=1.0
  out "Flow Valve % Closed":dbl format="%#.1f %%"
  in  "Flow Valve % Closed Cmd":dbl caption="Flow Valve % Closed" min=0.0 max=100.0 step=1.0
  out "Recirc Valve % Closed":dbl format="%#.1f %%"
  in  "Recirc Valve % Closed Cmd":dbl caption="Recirc Valve % Closed" min=0.0 max=100.0 step=1.0
  out "Pump Frequency [Hz]":dbl format="%#.1f Hz"
  in  "Pump Frequency Cmd [Hz]":dbl caption="Pump Frequency [Hz]" min=-1.0 max=76.5 step=1.0
  in  "Vent Valve":bool
  in  "Drive Air Enable":bool
  in  "Monitoring loop period (ms)":u32=200 caption="Loop Period (ms)" format="%.0f ms"
  in  "Exit":bool
  in  "Controller\nAddress":string="169.254.66.100"
  in  "File Name":string="SuNLaMP_%Y%m%d_%H%"
  in  "Data Folder Path":path=path "C:/LabView/Data"
  in  "Record?":bool
  in  "Settings Tab":T1(tab)=enum."RT Diagnostics"
  out "Recup Hot Inlet Pressure [psig]":dbl format="%#.1f psig"
  out "Recup Cold Inlet Pressure [psig]":dbl format="%#.1f psig"
  out "Heater Inlet Pressure [psig]":dbl format="%#.1f psig"
  out "Recup Hot dP [psid]":dbl format="%#.1f psid"
  out "Recup Cold dP [psid]":dbl format="%#.1f psid"
  out "Heater dP [psid]":dbl format="%#.1f psid"
  out "Heater Outlet Temperature [F]":dbl format="%#.1f F"
  out "Recup Hot Inlet Temperature [F]":dbl format="%#.1f F"
  out "Heater Inlet Temperature [F]":dbl format="%#.1f F"
  out "Recup Cold Outlet Temperature [F]":dbl format="%#.1f F"
  out "Recup Hot Outlet Temperature [F]":dbl format="%#.1f F"
  out "Recup Cold Inlet Temperature [F]":dbl format="%#.1f F"
  out "Water Outlet Temperature [F]":dbl caption="Water Outlet Temperature [F}" format="%#.1f F"
  out "Pump Outlet Temperature [F]":dbl format="%#.1f F"
  out "Water Inlet Pressure [psig]":dbl format="%#.1f psig"
  out "Water Outlet Pressure [psig]":dbl format="%#.1f psig"
  out "Water Inlet Temperature [F]":dbl caption="Water Inlet Temperature [F}" format="%#.1f F"
  out "Cooler Outlet Temperature [F]":dbl caption="Cooler Outlet Temperature [F}" format="%#.1f F"
  out "Water Flow Rate [gpm]":dbl format="%#.1f gpm"
  out "Pump Inlet Temperature [F]":dbl caption="Cooler CO2 In [F]" format="%#.1f F"
  out "Recup Cold Inlet Density [kg|m^3]":dbl caption="Density [g/cm^3]" format="%#_4f kg/m^3"
  out "Flow Rate [kg|s]":dbl format="%#_3g kg/s"
  out "Cooler Inlet Temperature [F]":dbl caption="Cooler CO2 In [F]" format="%#.1f F"
  out "Cooler CO2 Inlet Pressure [psig]":dbl caption="Pump" format="%#.1f psig"
  out "Inlet Filter dP [psid]":dbl caption="Return Filter dP [psid]" format="%#.1f psid"
  out "Cooler CO2 dP [psid]":dbl caption="Cooler dP [psid]" format="%#.1f psid"
  out "Outlet Filter dP [psid]":dbl caption="Outlet Filter and Flowmeter dp [psid]" format="%#.1f psid"
  out "Pump Outlet Pressure [psig]":dbl caption="Cooler CO2 Out [F]" format="%#.1f psig"
  out "Pump dP [psid]":dbl format="%#.1f psid"
  out "Pump Outlet Density [kg|m3]":dbl caption="Density [g/cm^3]" format="%#_4f kg/m^3"
  out "Pump Flow Rate [kg|s]":dbl caption="Flow Rate [kg/s]" format="%#_3g kg/s"
  in  "dPs":string="Recup Cold dP [psid]\nRecup Hot dP [psid]\nReturn Filter dP [psid]\nOutlet Filter dP [psid]\nHeater dP [psid]\nCooler CO2 dP [psid]\nPump dP [psid]\nWater Inlet Pressure [psig]\nWater Outlet Pressure [psig]\nHXer dP [psid]"
  in  "Temps":string="Recup Cold Outlet Temperature [F]\nRecup Hot Inlet Temperature [F]\nPump Outlet Temperature [F]\nPump Inlet Temperature [F]\nCooler Outlet Temperature [F]\nCooler Inlet Temperature [F]\nWater Inlet Temperature [F]\nWater Outlet Temperature [F]\nRecup Hot Outlet Temperature [F]\nRecup Cold Inlet Temperature [F]\nHeater Inlet Temperature [F]"
  in  "Pressures":string="Recup Cold Inlet Pressure [psig]\nRecup Hot Inlet Pressure [psig]\nHeater Inlet Pressure [psig]\nCooler CO2 Inlet Pressure [psig]\nPump Outlet Pressure [psig]\nHXer Inlet Pressure [psig]"
  out "Chart 1":waveform(dbl)[](graph)=[{"t0"=timestamp(3629387256.9663014 s since 1904-01-01), "dt"=1.0, "Y"=[-1.0576147437095735], "attributes"=variant("NI_ChannelName"=variant(string "Recup Cold Inlet Pressure [psig]"))}, {"t0"=timestamp(3629387256.9663014 s since 1904-01-01), "dt"=1.0, "Y"=[61.70975503325454], "attributes"=variant("NI_ChannelName"=variant(string "Recup Cold Outlet Temperature [F]"))}, {"t0"=timestamp(3629387256.9663014 s since 1904-01-01), "dt"=1.0, "Y"=[-0.03010556101799148], "attributes"=variant("NI_ChannelName"=variant(string "Recup Cold dP [psid]"))}, {"t0"=timestamp(3629387256.9663014 s since 1904-01-01), "dt"=1.0, "Y"=[0.0], "attributes"=variant("NI_ChannelName"=variant(string "Pump Frequency Cmd [Hz]"))}]
  out "message log":string
  out "System Status":string
  in  "Number of Buffer Files (48)":i32=48
  in  "Buffer Write Limit (36000)":i32=36000
  out "Connected?":bool
  in  "Connect to Controller":bool
  out "indicator labels":string[](array[string])
  out "control labels":string[](array[string])
  out "indicator class names":string[](array[string])
  out "control refnums":refnum<vi>[](array[refnum])
  out "indicator refnums":refnum<vi>[](array[refnum])
  out "control class names":string[](array[string])
  out "indicators error":errorcluster
  out "all data":cluster{"String":string, "Numeric":dbl}[](array[cluster])
  out "error out":errorcluster
  out "Raw Data":T2(array[cluster])
  in  "Formulas":string[](array[string])=["Flow Rate [gpm]=Flow Rate [kg/s]/Density [kg/m^3]*15850", "Head Rise [ft] = Pump dP [psid] * 2.307", "Dead Head [psig] = Regulated Pressure [psig] + Drive Air Pressure Cmd [psig] * 60"]
  # "Controls"
  # "System Controls"
  # "Data Log"
  # "System Settings"
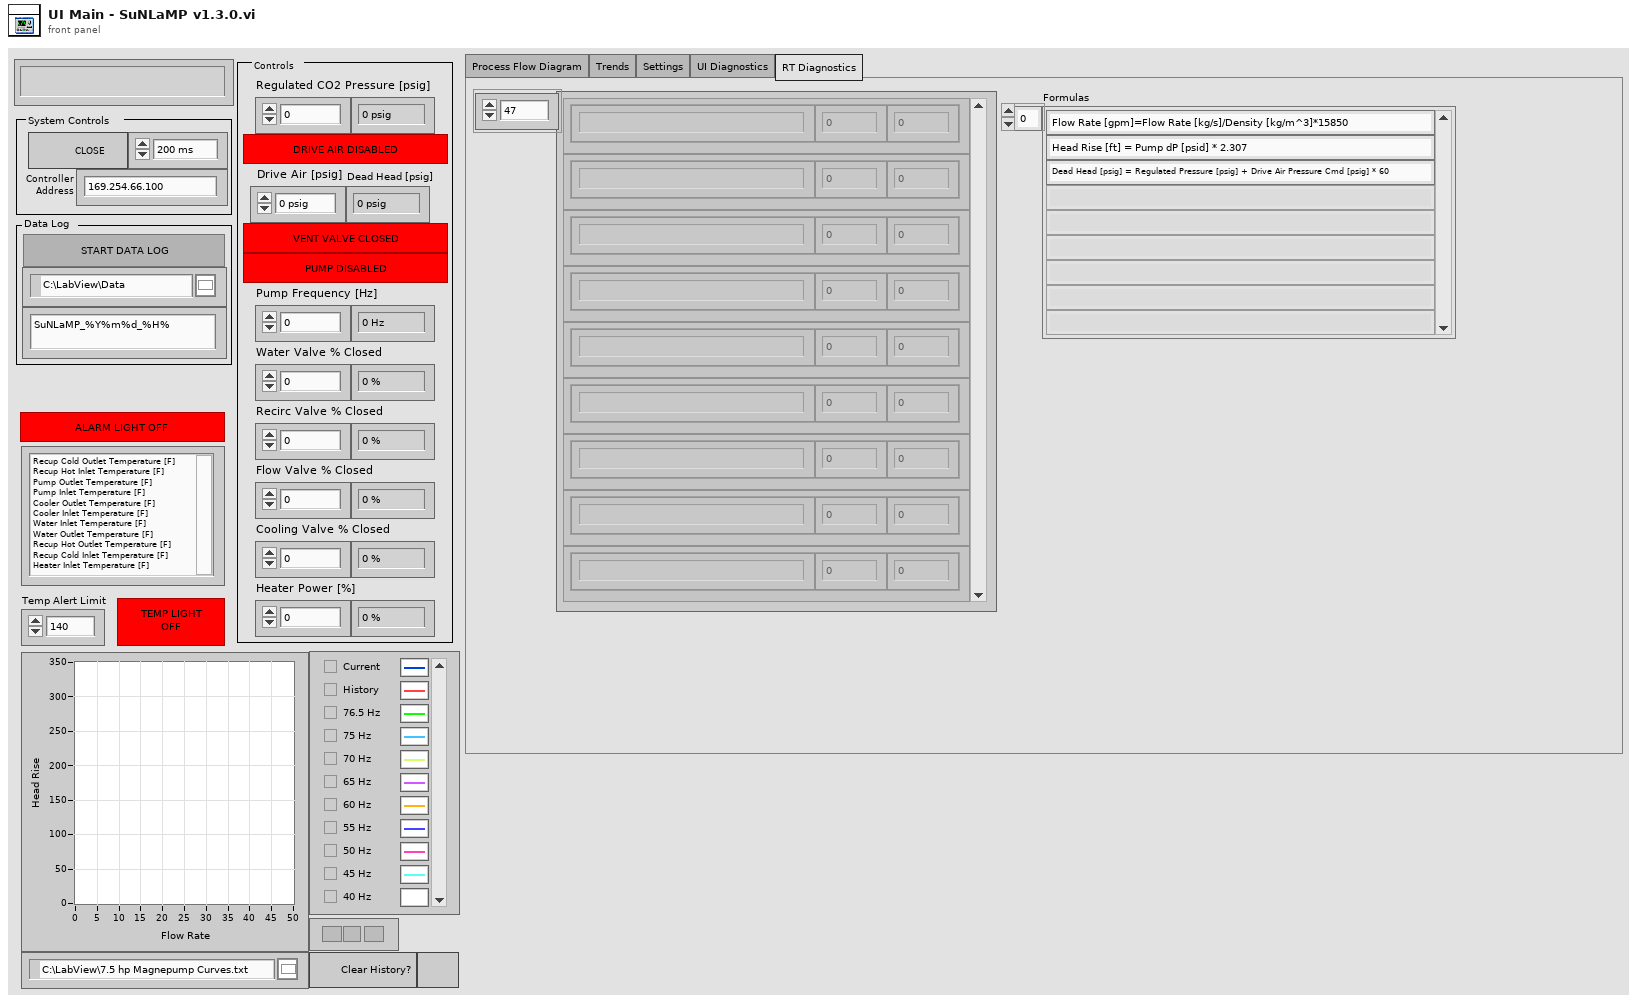
[diagram p1: front panel]
types:
  T1 = enum32{"Process Flow Diagram", "Trends", "Settings", "UI Diagnostics", "RT Diagnostics"}
  T2 = cluster{"String":string, "Double":dbl, "code":i32}[]
  T3 = typedef "Message Queue.lvlib/All Message Queues.ctl" = cluster{"UI":refnum<queue>}
  T4 = enum16{"flow & head", "head & speed", "flow & speed"}
  T5 = enum16{"load plot settings", "save plot settings", "update plot names", "update plot values", "clear plot histories"}
  T6 = enum8{"Enabled", "Disabled", "Disabled and Grayed Out"}
  T7 = cluster{"Message":string, "Message Data":variant}
  T8 = typedef "Variable References.ctl" = cluster{"CPU Usage":refnum<k21>, "Contiguous Memory":refnum<k21>, "Control Mode":refnum<k21>, "Control Loop Period":refnum<k21>, "Input Values":refnum<k21>, "Output Values":refnum<k21>}
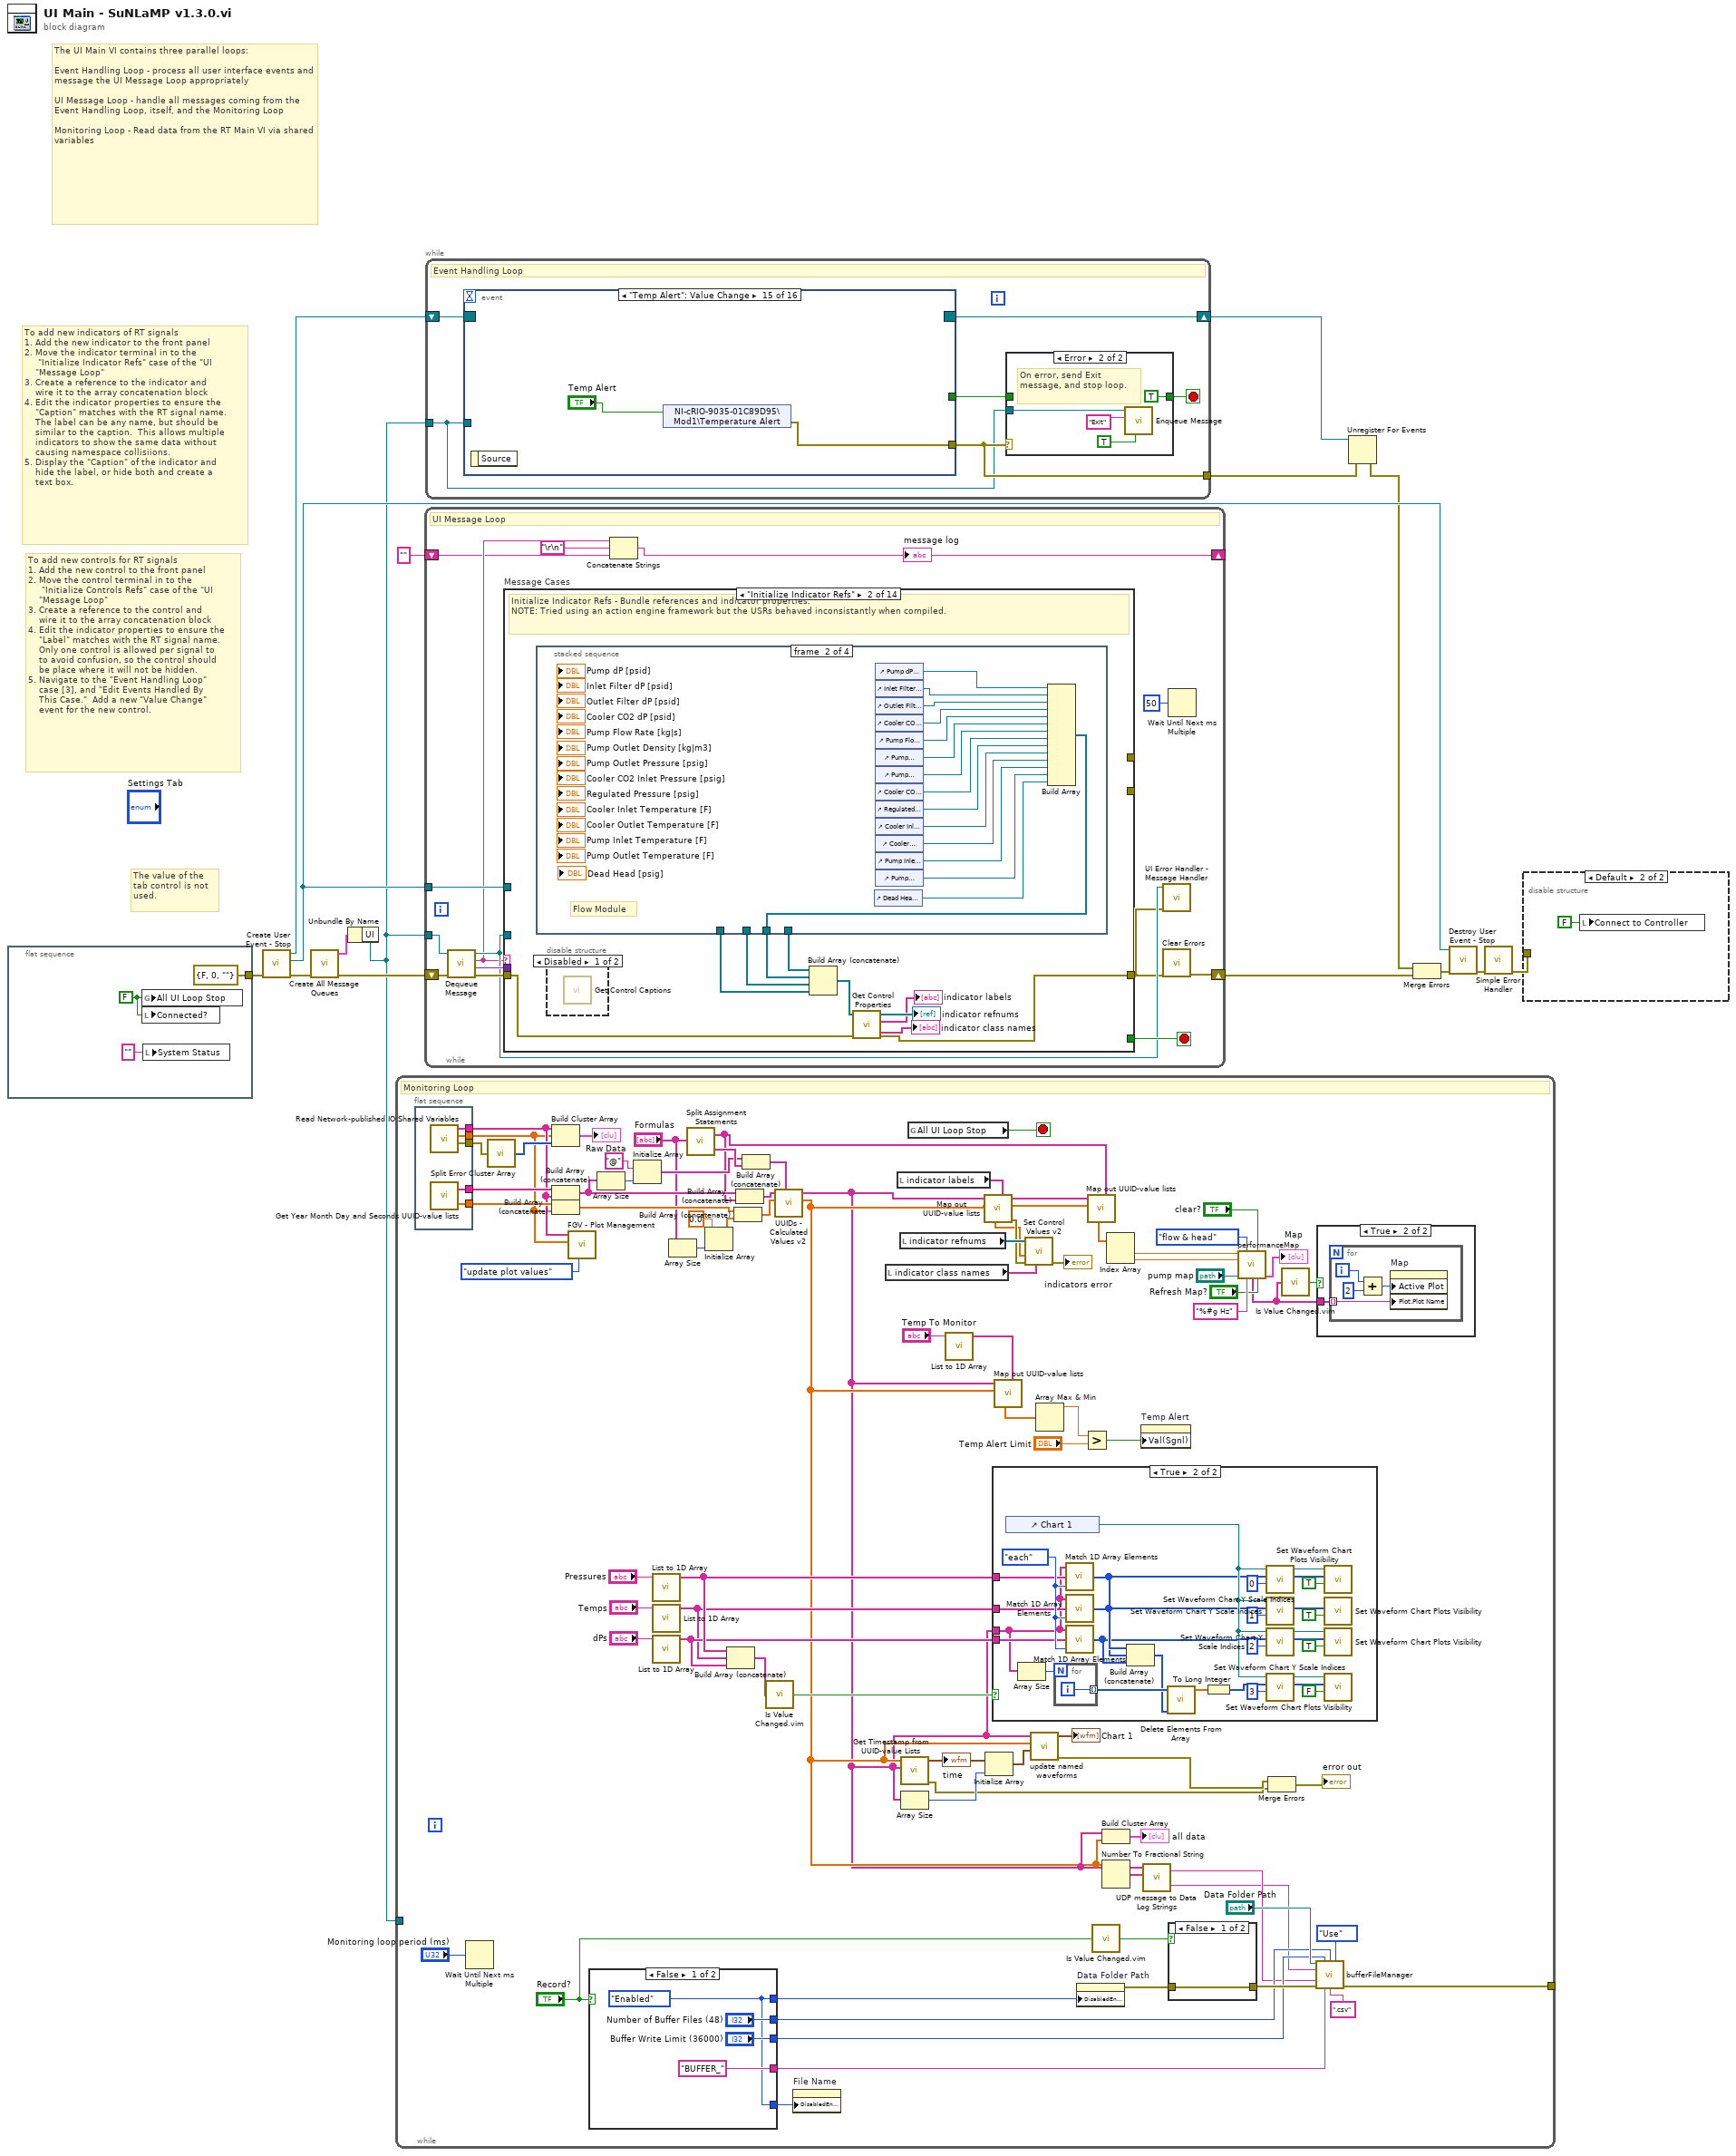
[diagram p0: block diagram]
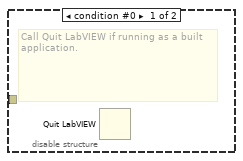
[diagram p2: hidden frame]
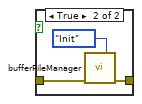
[diagram p5: hidden frame]
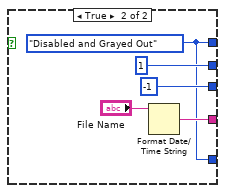
[diagram p6: hidden frame]
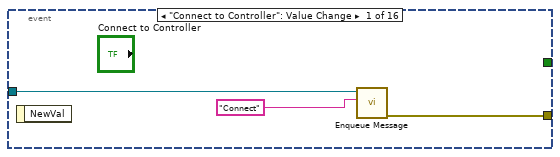
[diagram p8: hidden frame]
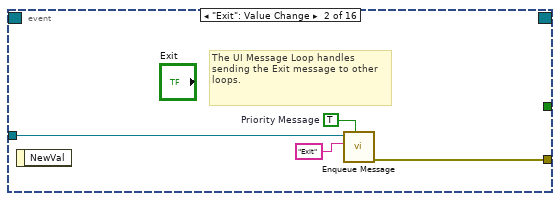
[diagram p9: hidden frame]
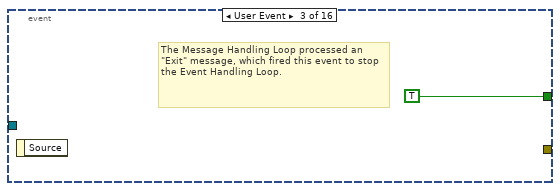
[diagram p10: hidden frame]
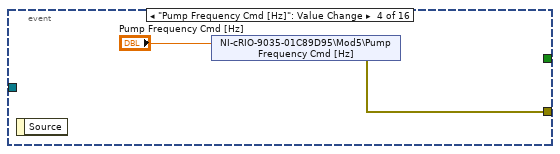
[diagram p11: hidden frame]
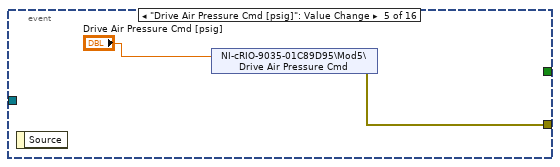
[diagram p12: hidden frame]
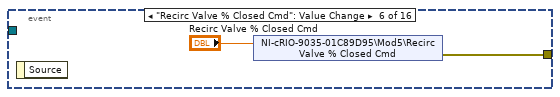
[diagram p13: hidden frame]
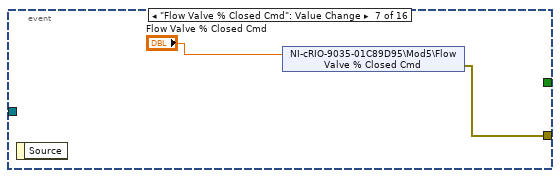
[diagram p14: hidden frame]
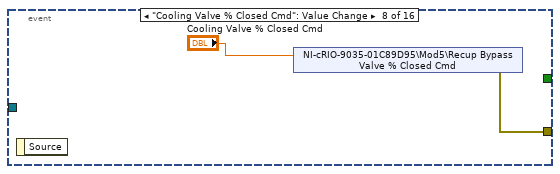
[diagram p15: hidden frame]
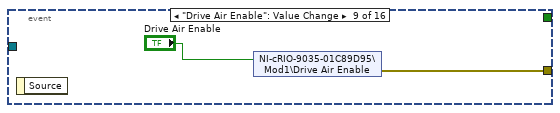
[diagram p16: hidden frame]
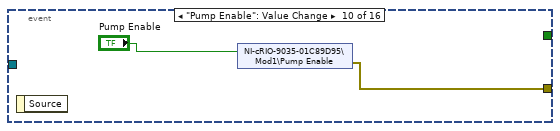
[diagram p17: hidden frame]
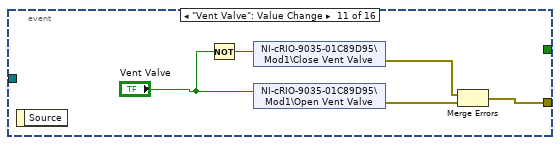
[diagram p18: hidden frame]
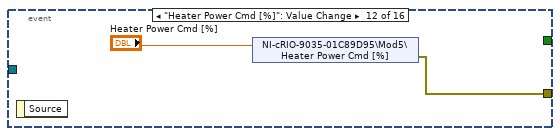
[diagram p19: hidden frame]
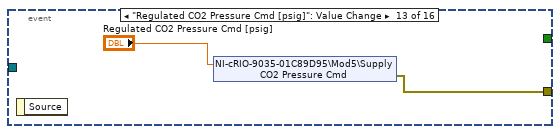
[diagram p20: hidden frame]
diagram:
  # "To add new controls for RT signals\n1. Add the new control to the front panel\n2. Move the control terminal in to the \n     \"Initialize Controls Refs\" case of the \"UI \n    \"Message Loop\"\n3. Create a reference to the control and \n    wire it to the array concatenation block\n4. Edit the indicator properties to ensure the \n    \"Label\" matches with the RT signal name.\n    Only one control is allowed per signal to \n    to avoid confusion, so the control should\n    be place where it will not be hidden.\n5. Navigate to the \"Event Handling Loop\" \n    case [3], and \"Edit Events Handled By \n    This Case.\"  Add a new \"Value Change\" \n    event for the new control."
  # "To add new indicators of RT signals\n1. Add the new indicator to the front panel\n2. Move the indicator terminal in to the \n     \"Initialize Indicator Refs\" case of the \"UI \n    \"Message Loop\"\n3. Create a reference to the indicator and \n    wire it to the array concatenation block\n4. Edit the indicator properties to ensure the \n    \"Caption\" matches with the RT signal name.\n    The label can be any name, but should be \n    similar to the caption.  This allows multiple \n    indicators to show the same data without \n    causing namespace collisiions.\n5. Display the \"Caption\" of the indicator and \n    hide the label, or hide both and create a \n    text box."
  # "The UI Main VI contains three parallel loops:\n\nEvent Handling Loop - process all user interface events and message the UI Message Loop appropriately\n\nUI Message Loop - handle all messages coming from the Event Handling Loop, itself, and the Monitoring Loop\n\nMonitoring Loop - Read data from the RT Main VI via shared variables"
  # "The value of the tab control is not used."
  n1 = flat-sequence {
    tunnel: [errorcluster {"status"=FALSE, "code"=0, "source"=""} ("error in (no error)")] -> w4
    frame #0 {
      w16 = FALSE
      n2 = global write "Global - All UI Loop Stop.vi" "All UI Loop Stop"(w16) -> ()
      n3 = local write "Connected?"(w16) -> ()
      n4 = local write "System Status"("" ("System Status")) -> ()
    }
  }
  n5 = call "Create User Event - Stop.vi"("error in (no error)"=w4) -> ("error out"=w10:errorcluster, "User Event - Stop"=w11:refnum<user-event>, "Stop Event Registration Refnum"=w12:refnum<event-registration>)  [unwired: 8 in]
  n6 = call "Create All Message Queues.vi"("error in (no error)"=w10) -> ("error out"=w8:errorcluster, "Message Queues out"=w9:T3)  [unwired: 9 in]
  n7 = Unbundle By Name(w9) -> ("UI"=w1:refnum<queue>)
  n8 = while {
    tunnel: [w99] -> _
    tunnel: w1 -> [_]
    stop <- w101 stop-if-true
    # "Monitoring Loop"
    n9 = flat-sequence {
      tunnel: [w137] -> w86
      tunnel: [w136] -> w71
      tunnel: [w135] -> w56
      tunnel: [w134] -> w80
      tunnel: [w133] -> w79
      frame #0 {
        n10 = call "Read Network-published IO Shared Variables.vi"() -> ("channel errors"=w137:errorcluster[], "data"=w135:dbl[], "UUIDs"=w136:string[])  [unwired: 9 in]
        n11 = call "Get Year Month Day and Seconds UUID-value lists.vi"() -> ("values"=w133:dbl[], "UUIDs"=w134:string[])  [unwired: 2 in]
      }
    }
    n12 = Wait Until Next ms Multiple(millisecond multiple="Monitoring loop period (ms)") -> ()  [unwired: 1 out]
    n13 = call "Split Error Cluster Array.vi"("Error cluster array"=w86) -> ("codes"=w85:i32[])  [unwired: 2 out]
    n14 = Build Cluster Array(w71, w56, w85) -> (→"Raw Data":T2)
    n15 = Build Array (concatenate)(w80, w71) -> (w66:string[])
    n16 = Build Array (concatenate)(w79, w56) -> (w61:dbl[])
    n17 = call "FGV - Plot Management.vi"("Mode"=T5."update plot values", "Values"=w56, "UUIDs"=w71) -> ()  [unwired: 8 in, 1 out]
    n18 = case shown="False" "Record?" {
      tunnel: [w142 w146] -> w94
      tunnel: ["BUFFER_" ("date/time string") w150] -> w91
      tunnel: ["Number of Buffer Files (48)" 1 ("Number of Files (7)")] -> w89
      tunnel: ["Buffer Write Limit (36000)" -1 ("Write Limit (6000 writes)")] -> w90
      tunnel: [w142 w146] -> w87
      frame False {
        w142 = T6."Enabled" ("Disabled")
      }
      frame True {
        w146 = T6."Disabled and Grayed Out" ("Disabled")
        n19 = Format Date/Time String(time format string (%c)="File Name") -> (date/time string=w150:string)  [unwired: 2 in]
      }
    }
    n20 = Array Size(array=w66) -> (size(s)=w70:i32)
    n21 = Initialize Array("@", w70) -> (w67:string[])
    n22 = call "List to 1D Array.vi"("List String"="Pressures") -> ("1D Array"=w30:string[])  [unwired: 10 in]
    n23 = call "List to 1D Array.vi"("List String"="Temps") -> ("1D Array"=w27:string[])  [unwired: 10 in]
    n24 = call "List to 1D Array.vi"("List String"="dPs") -> ("1D Array"=w29:string[])  [unwired: 10 in]
    n25 = Array Size(array="Formulas") -> (size(s)=w59:i32)
    n26 = call "Split Assignment Statements.vi"("Formulas"="Formulas") -> ("Assigned Vars"=w53:string[], "Expressions"=w68:string[])
    n27 = Initialize Array(0.0, w59) -> (w57:dbl[])
    n28 = Build Array (concatenate)(w30, w27, w29) -> (w31:string[])
    n29 = Build Array (concatenate)(w61, w57) -> (w62:dbl[])
    n30 = Build Array (concatenate)(w66, w53) -> (w65:string[])
    n31 = Build Array (concatenate)(w67, w68) -> (w64:string[])
    n32 = call "Is Value Changed.vim"("value"=w31) -> ("changed or first call?"=w35:bool)
    n33 = call "UUIDs - Calculated Values v2.vi"("Expressions"=w64, "values in"=w62, "UUIDs in"=w65) -> ("values out"=w26:dbl[], "UUIDs out"=w25:string[])  [unwired: 6 in, 1 out]
    n34 = property on="File Name" class="Str"("DisabledEnum"=w87) -> ()  [unwired: 2 in, 2 out]
    n35 = local read "indicator class names"() -> (w76:string[])
    n36 = local read "indicator labels"() -> (w78:string[])
    n37 = local read "indicator refnums"() -> (w77:refnum<vi>[])
    n38 = call "Get Timestamp from UUID-value Lists.vi"("UUIDs"=w25, "Values"=w26) -> ("error out"=w37:errorcluster, "time stamp"=w41:timestamp)  [unwired: 8 in]
    "time" <- w41
    n39 = Array Size(array=w25) -> (size(s)=w40:i32)
    n40 = global read "Global - All UI Loop Stop.vi" "All UI Loop Stop"() -> (w101:bool)
    n41 = call "List to 1D Array.vi"("List String"="Temp To Monitor") -> ("1D Array"=w19:string[])  [unwired: 10 in]
    n42 = call "Map out UUID-value lists.vi"("UUIDs to extract"=w78, "values in"=w26, "UUIDs in"=w25) -> ("error out"=w75:errorcluster, "values out"=w54:dbl[], "UUIDs out"=w55:string[], "values extracted"=w73:dbl[])  [unwired: 4 in, 1 out]
    n43 = Initialize Array(w41, w40) -> (w39:timestamp[])
    n44 = case shown="True" w35 {
      tunnel: w25 -> [_ w113]
      tunnel: w30 -> [_ w117]
      tunnel: w27 -> [_ w116]
      tunnel: w29 -> [_ w115]
      frame False {
      }
      frame True {
        w118 = enum16{"any", "each"}."each" ("mode (any)")
        n45 = control-ref of="Chart 1"() -> (w114:refnum<vi>)
        n46 = Array Size(array=w113) -> (size(s)=w112:i32)
        n47 = for {
          N: w112 -> [_]
          tunnel: [w127] -> w108 mode=indexing
          i -> [w127]
        }
        n48 = call-poly "Match 1D Array Elements.vi"("mode (any)"=w118, "elements (none)"=w117, "1D Array"=w113) -> ("indices"=w111:i32[])
        n49 = call-poly "Match 1D Array Elements.vi"("mode (any)"=w118, "elements (none)"=w116, "1D Array"=w113) -> ("indices"=w110:i32[])
        n50 = call-poly "Match 1D Array Elements.vi"("mode (any)"=w118, "elements (none)"=w115, "1D Array"=w113) -> ("indices"=w109:i32[])
        n51 = Build Array (concatenate)(w111, w110, w109) -> (w107:i32[])
        n52 = call-poly "Delete Elements From Array.vi"("indices (none)"=w107, "1D Array"=w108) -> ("array w/ subset deleted"=w103:dbl[])  [unwired: 8 in, 1 out]
        n53 = To Long Integer(number=w103) -> (32bit integer=w102:i32[])
        n54 = call "Set Waveform Chart Y Scale Indices.vi"("YScaleIdxs"=u32 0, "Active Plot"=w111, "WaveformChart in"=w114) -> ("WaveformChart out"=w123:refnum<vi>)  [unwired: 7 in, 1 out]
        n55 = call "Set Waveform Chart Y Scale Indices.vi"("YScaleIdxs"=u32 1, "Active Plot"=w110, "WaveformChart in"=w114) -> ()  [unwired: 7 in, 2 out]
        n56 = call "Set Waveform Chart Y Scale Indices.vi"("YScaleIdxs"=u32 2, "Active Plot"=w109, "WaveformChart in"=w114) -> ("WaveformChart out"=w126:refnum<vi>)  [unwired: 7 in, 1 out]
        n57 = call "Set Waveform Chart Y Scale Indices.vi"("YScaleIdxs"=u32 3, "Active Plot"=w102, "WaveformChart in"=w114) -> ("WaveformChart out"=w106:refnum<vi>)  [unwired: 7 in, 1 out]
        n58 = call "Set Waveform Chart Plots Visibility.vi"("Plot.Visible"=TRUE, "Active Plot"=w111, "WaveformChart in"=w123) -> ()  [unwired: 7 in, 2 out]
        n59 = call "Set Waveform Chart Plots Visibility.vi"("Plot.Visible"=TRUE, "Active Plot"=w110) -> ()  [unwired: 8 in, 2 out]
        n60 = call "Set Waveform Chart Plots Visibility.vi"("Plot.Visible"=TRUE, "Active Plot"=w109, "WaveformChart in"=w126) -> ()  [unwired: 7 in, 2 out]
        n61 = call "Set Waveform Chart Plots Visibility.vi"("Plot.Visible"=FALSE, "Active Plot"=w102, "WaveformChart in"=w106) -> ()  [unwired: 7 in, 2 out]
      }
    }
    n62 = call "Map out UUID-value lists.vi"("UUIDs to extract"=w19, "values in"=w26, "UUIDs in"=w25) -> ("values extracted"=w24:dbl[])  [unwired: 4 in, 4 out]
    n63 = call "Set Control Values v2.vi"("class names"=w76, "error in"=w75, "values"=w73, "refnums in"=w77) -> ("error out"=→"indicators error":errorcluster)  [unwired: 6 in, 1 out]
    n64 = call "update named waveforms.vi"("timestamps"=w39, "values"=w26, "names"=w25) -> ("error out"=w38:errorcluster, "waveforms out"=→"Chart 1":waveform(dbl)[])  [unwired: 7 in]
    n65 = Array Max & Min(array=w24) -> (max value=w23:dbl)  [unwired: 3 out]
    n66 = property on="Data Folder Path" class="Path"("DisabledEnum"=w94) -> (error out=w93:errorcluster)  [unwired: 2 in, 1 out]
    n67 = Greater?(x=w23, y="Temp Alert Limit") -> (0:w21:bool)
    n68 = call "Map out UUID-value lists.vi"("UUIDs to extract"=w53, "values in"=w54, "UUIDs in"=w55) -> ("values extracted"=w52:dbl[])  [unwired: 4 in, 4 out]
    n69 = call "Is Value Changed.vim"("value"="Record?") -> ("changed or first call?"=w96:bool)
    n70 = Build Cluster Array(w25, w26) -> (→"all data":cluster{string, "Numeric":dbl}[])
    n71 = Number To Fractional String(number=w26) -> (F-format string=w81:string[])  [unwired: 3 in]
    n72 = Index Array(array=w52) -> (element #1=w43:dbl, element #2=w42:dbl)  [unwired: 2 in]
    n73 = property on="Temp Alert" class="Bool (strict)"("Val(Sgnl)"=w21) -> ()  [unwired: 2 in, 2 out]
    n74 = call "UDP message to Data Log Strings.vi"("Values"=w81, "UUIDs"=w25) -> ("Data String"=w82:string, "Header String"=w83:string)  [unwired: 2 in]
    n75 = case shown="False" w96 {
      tunnel: w93 -> [w138 w141]
      tunnel: [w138 w139] -> w92
      frame False {
      }
      frame True {
        n76 = call "bufferFileManager.vi"("Mode (Use)"=enum16{"Init", "Use"}."Init", "Error In (no error)"=w141) -> ("Error Out"=w139:errorcluster)  [unwired: 10 in, 3 out]
      }
    }
    n77 = call "performanceMap.vi"("Flow"=w43, "mode"=T4."flow & head", "clear?"="clear?", "Head"=w42, "file path (dialog if empty)"="pump map", "label format"="%#g Hz", "reload?"="Refresh Map?") -> ("z labels"=w44:string[], "Performance Map"=→"Map":cluster{dbl[], dbl[]}[])  [unwired: 4 in, 3 out]
    n78 = Merge Errors(w38, w37) -> (→"error out":errorcluster)
    n79 = call "Is Value Changed.vim"("value"=w44) -> ("changed or first call?"=w46:bool)
    n80 = call "bufferFileManager.vi"("Base Path (C:\\)"="Data Folder Path", "Write Limit (6000 writes)"=w90, "Number of Files (7)"=w89, "Mode (Use)"=enum16{"Init", "Use"}."Use", "Data Byte String (empty string)"=w82, "Header Byte String (empty string)"=w83, "Error In (no error)"=w92, "File Name Template (BUFFER_)"=w91, "File Extension (none)"=".csv") -> ("Error Out"=w99:errorcluster)  [unwired: 3 in, 3 out]
    n81 = case shown="True" w46 {
      tunnel: w44 -> [_ w128]
      frame False {
      }
      frame True {
        n82 = for {
          tunnel: w128 -> [w130] mode=indexing
          i -> [w132]
          n83 = Add(x=w132, y=2) -> (x+y=w129:i32)
          n84 = property on="Map" class="XYGraph (strict)"("Active Plot"=w129, "Plot.Plot Name"=w130) -> ()  [unwired: 2 in, 2 out]
        }
      }
    }
  }
  n85 = while {
    tunnel: w1 -> [w159]
    tunnel: w11 -> [w163]
    shift-right: [w156] -> w15
    shift-left: w8 -> [w162]
    shift-right: [w152] -> _
    shift-left: "" -> [w153]
    stop <- w164 stop-if-true
    # "UI Message Loop"
    n86 = call "Dequeue Message.vi"("error in (no error)"=w162, "Message Queue"=w159) -> ("error out"=w161:errorcluster, "Message Data"=w160:variant, "Message"=w155:string, "dup Message Queue"=w158:refnum<queue>)  [unwired: 6 in]
    n87 = case "Message Cases" shown="\"Initialize Indicator Refs\"" w155 {
      selector: w155 -> [_ _ _ _ _ _ _ w281 w297 _ _ _ _ w366]
      tunnel: w158 -> [w169 _ _ _ w243 w258 _ _ w301 _ w346 _ _ _]
      tunnel: w161 -> [w170 w182 w229 w237 w245 w259 w269 w282 w311 w330 w350 w359 w362 _]
      tunnel: [w167 w181 w228 w236 w242 w257 w268 w279 w312 w329 w351 w360 w361 w364] -> w157
      tunnel: [_ _ _ _ _ _ _ _ _ _ TRUE _ _ _] -> w164
      tunnel: w160 -> [_ _ _ _ _ _ _ w280 w309 w328 _ _ _ _]
      tunnel: w163 -> [_ _ _ _ _ _ _ _ _ _ w349 _ _ _]
      tunnel: [_ _ _ _ _ _ _ _ _ _ w339 _ _ _] -> _
      tunnel: [_ _ _ _ _ _ _ _ _ _ w338 _ _ _] -> _
      frame "Initialize" {
        w165 = 0.0 ("Value (Signaling)")
        w166 = FALSE ("Value (Signaling)")
        w168 = string[] ["Initialize Indicator Refs", "Initialize Controls Refs"]  # Initializiation Steps
        # "Initialize - Perform a series of UI initialization steps\nNOTE: These must be added first to minimize the risk of a race condition with user/monitored events."
        n88 = property on="Pump Enable" class="Bool (strict)"("Val(Sgnl)"=w166) -> ()  [unwired: 2 in, 2 out]
        n89 = property on="Vent Valve" class="Bool (strict)"("Val(Sgnl)"=w166) -> ()  [unwired: 2 in, 2 out]
        n90 = property on="Drive Air Enable" class="Bool (strict)"("Val(Sgnl)"=w166) -> ()  [unwired: 2 in, 2 out]
        n91 = property on="Pump Frequency Cmd [Hz]" class="DigNum (strict)"("Val(Sgnl)"=w165) -> ()  [unwired: 2 in, 2 out]
        n92 = property on="Regulated CO2 Pressure Cmd [psig]" class="DigNum (strict)"("Val(Sgnl)"=w165) -> ()  [unwired: 2 in, 2 out]
        n93 = property on="Drive Air Pressure Cmd [psig]" class="DigNum (strict)"("Val(Sgnl)"=w165) -> ()  [unwired: 2 in, 2 out]
        n94 = property on="Heater Power Cmd [%]" class="DigNum (strict)"("Val(Sgnl)"=w165) -> ()  [unwired: 2 in, 2 out]
        n95 = for {
          tunnel: w169 -> [w173]
          tunnel: w168 -> [w172] mode=indexing
          shift-right: [w171] -> w167
          shift-left: w170 -> [w174]
          n96 = call "Enqueue Message.vi"("error in (no error)"=w174, "Message"=w172, "Message Queue"=w173) -> ("error out"=w171:errorcluster)  [unwired: 7 in, 1 out]
        }
      }
      frame "Initialize Indicator Refs" {
        # "Initialize Indicator Refs - Bundle references and indicator properties.\nNOTE: Tried using an action engine framework but the USRs behaved inconsistantly when compiled."
        n97 = stacked-sequence {
          tunnel: [w185 _ _ _] -> w178
          tunnel: [_ w195 _ _] -> w177
          tunnel: [_ _ w207 _] -> w176
          tunnel: [_ _ _ w225] -> w175
          frame #0 {
            # "AO"
            n98 = control-ref of="Pump Frequency [Hz]"() -> (w191:refnum<vi>)
            n99 = control-ref of="Heater Power [%]"() -> (w190:refnum<vi>)
            n100 = control-ref of="Recirc Valve % Closed"() -> (w189:refnum<vi>)
            n101 = control-ref of="Flow Valve % Closed"() -> (w188:refnum<vi>)
            n102 = control-ref of="Cooling Valve % Closed"() -> (w187:refnum<vi>)
            n103 = control-ref of="Water Valve % Closed"() -> (w186:refnum<vi>)
            n104 = Build Array(w191, w190, w189, w188, w187, w186) -> (w185:refnum<vi>[])
          }
          frame #1 {
            # "Flow Module"
            n105 = control-ref of="Dead Head [psig]"() -> (w194:refnum<vi>)
            n106 = control-ref of="Pump dP [psid]"() -> (w206:refnum<vi>)
            n107 = control-ref of="Inlet Filter dP [psid]"() -> (w205:refnum<vi>)
            n108 = control-ref of="Outlet Filter dP [psid]"() -> (w204:refnum<vi>)
            n109 = control-ref of="Cooler CO2 dP [psid]"() -> (w203:refnum<vi>)
            n110 = control-ref of="Pump Flow Rate [kg|s]"() -> (w202:refnum<vi>)
            n111 = control-ref of="Pump Outlet Density [kg|m3]"() -> (w201:refnum<vi>)
            n112 = control-ref of="Pump Outlet Pressure [psig]"() -> (w200:refnum<vi>)
            n113 = control-ref of="Cooler CO2 Inlet Pressure [psig]"() -> (w199:refnum<vi>)
            n114 = control-ref of="Regulated Pressure [psig]"() -> (w198:refnum<vi>)
            n115 = control-ref of="Cooler Inlet Temperature [F]"() -> (w197:refnum<vi>)
            n116 = control-ref of="Cooler Outlet Temperature [F]"() -> (w196:refnum<vi>)
            n117 = control-ref of="Pump Inlet Temperature [F]"() -> (w193:refnum<vi>)
            n118 = control-ref of="Pump Outlet Temperature [F]"() -> (w192:refnum<vi>)
            n119 = Build Array(w206, w205, w204, w203, w202, w201, w200, w199, w198, w197, w196, w193, w192, w194) -> (w195:refnum<vi>[])
          }
          frame #2 {
            # "Water System"
            n120 = control-ref of="Water Flow Rate [gpm]"() -> (w212:refnum<vi>)
            n121 = control-ref of="Water Inlet Pressure [psig]"() -> (w211:refnum<vi>)
            n122 = control-ref of="Water Outlet Pressure [psig]"() -> (w210:refnum<vi>)
            n123 = control-ref of="Water Outlet Temperature [F]"() -> (w209:refnum<vi>)
            n124 = control-ref of="Water Inlet Temperature [F]"() -> (w208:refnum<vi>)
            n125 = Build Array(w212, w211, w210, w209, w208) -> (w207:refnum<vi>[])
          }
          frame #3 {
            # "Recuperator"
            n126 = control-ref of="Recup Cold Inlet Density [kg|m^3]"() -> (w227:refnum<vi>)
            n127 = control-ref of="Flow Rate [kg|s]"() -> (w226:refnum<vi>)
            n128 = control-ref of="Recup Cold Inlet Temperature [F]"() -> (w224:refnum<vi>)
            n129 = control-ref of="Heater Inlet Pressure [psig]"() -> (w223:refnum<vi>)
            n130 = control-ref of="Recup Cold Inlet Pressure [psig]"() -> (w222:refnum<vi>)
            n131 = control-ref of="Recup Hot Inlet Pressure [psig]"() -> (w221:refnum<vi>)
            n132 = control-ref of="Heater dP [psid]"() -> (w220:refnum<vi>)
            n133 = control-ref of="Recup Cold dP [psid]"() -> (w219:refnum<vi>)
            n134 = control-ref of="Recup Hot dP [psid]"() -> (w218:refnum<vi>)
            n135 = control-ref of="Recup Hot Outlet Temperature [F]"() -> (w217:refnum<vi>)
            n136 = control-ref of="Recup Cold Outlet Temperature [F]"() -> (w216:refnum<vi>)
            n137 = control-ref of="Heater Inlet Temperature [F]"() -> (w215:refnum<vi>)
            n138 = control-ref of="Recup Hot Inlet Temperature [F]"() -> (w214:refnum<vi>)
            n139 = control-ref of="Heater Outlet Temperature [F]"() -> (w213:refnum<vi>)
            n140 = Build Array(w227, w226, w224, w223, w222, w221, w220, w219, w218, w217, w216, w215, w214, w213) -> (w225:refnum<vi>[])
          }
        }
        n141 = disable-structure shown="Disabled" {
          frame Disabled {
            n142 = call "Get Control Captions.vi"() -> ()  [unwired: 2 in, 2 out]
          }
          frame Enabled {
          }
        }
        n143 = Build Array (concatenate)(w178, w177, w176, w175) -> (w179:refnum<vi>[])
        n144 = call "Get Control Properties.vi"("error in"=w182, "refnums in"=w179) -> ("error out"=w181:errorcluster, "labels"=→"indicator labels":string[], "refnums out"=→"indicator refnums":refnum<vi>[], "class names"=→"indicator class names":string[])  [unwired: 4 in, 2 out]
      }
      frame "Initialize Controls Refs" {
        # "Initialize Manual Refs - Bundle references and manual control properties.\nNOTE: Tried using an action engine framework but the USRs behaved inconsistantly when compiled."
        n145 = disable-structure shown="Enabled" {
          disable-tunnel: w229 -> [w234 w235]
          disable-tunnel: [w233 w235] -> w228
          frame Disabled {
            # "ADD NEW CONTROLS HERE"
            n146 = call "Get Control Properties.vi"("error in"=w234) -> ("error out"=w233:errorcluster, "labels"=→"control labels":string[], "refnums out"=→"control refnums":refnum<vi>[], "class names"=→"control class names":string[])  [unwired: 5 in, 2 out]
          }
          frame Enabled {
          }
        }
      }
      frame "Disable Controls" {
        # "Disable all controls when not connected to the RT"
        n147 = disable-structure shown="Enabled" {
          disable-tunnel: w237 -> [w240 w241]
          disable-tunnel: [w238 w241] -> w236
          frame Disabled {
            n148 = local read "control refnums"() -> (w239:refnum<vi>[])
            n149 = call "Disable Controls.vi"("error in"=w240, "refnums in"=w239) -> ("error out"=w238:errorcluster)  [unwired: 8 in, 1 out]
          }
          frame Enabled {
          }
        }
      }
      frame "Connect" {
        # "Connect - Attempt to connect to both streams, and the variables, on the RT target.\nNOTE: Automatically enqueues \"Get Control Settings from RT\" on success and \"Disconnect UI\" on failure"
        n150 = disable-structure shown="Enabled" {
          disable-tunnel: w245 -> [w251 w256]
          disable-tunnel: "Controller\nAddress" -> [w250 _]
          disable-tunnel: w243 -> [w249 _]
          disable-tunnel: [w246 w256] -> w242
          frame Disabled {
            n151 = call "UI - Initiate Connection v2.vi"("error in (no error)"=w251, "Controller Address"=w250, "Message Queue"=w249) -> ("error out"=w247:errorcluster, "Connected?"=w248:bool)  [unwired: 7 in]
            "Connected?" <- w248
            n152 = case shown="True" w248 {
              tunnel: w247 -> [w252 w255]
              tunnel: [w252 w254] -> w246
              frame False {
              }
              frame True {
                n153 = property on="Controller\nAddress" class="Str"(error in=w255, "DisabledEnum"=T6."Disabled and Grayed Out" ("Disabled")) -> (error out=w254:errorcluster)  [unwired: 1 in, 1 out]
              }
            }
          }
          frame Enabled {
          }
        }
      }
      frame "Disconnect UI" {
        # "Disconnect UI - Something has gone wrong with the connection. Reinitialize the UI to its disconnected state."
        n154 = disable-structure shown="Enabled" {
          disable-tunnel: w259 -> [w265 w267]
          disable-tunnel: w258 -> [w264 _]
          disable-tunnel: [w261 w267] -> w257
          frame Disabled {
            w263 = FALSE ("Connected?")
            n155 = call "Enqueue Message.vi"("error in (no error)"=w265, "Message"="Disable Controls", "Message Queue"=w264) -> ("error out"=w262:errorcluster)  [unwired: 7 in, 1 out]
            n156 = local write "Connect to Controller"(w263) -> ()
            n157 = local write "Connected?"(w263) -> ()
            n158 = property on="Controller\nAddress" class="Str"(error in=w262, "DisabledEnum"=T6."Enabled" ("Disabled")) -> (error out=w261:errorcluster)  [unwired: 1 in, 1 out]
          }
          frame Enabled {
          }
        }
      }
      frame "Get Control Settings from RT" {
        # "Get Control Settings from RT - Send a command to the RT to retrieve all current control parameter values and send them back to the UI."
        n159 = disable-structure shown="Enabled" {
          disable-tunnel: w269 -> [w272 w278]
          disable-tunnel: [w271 w278] -> w268
          frame Disabled {
            n160 = local read "Connected?"() -> (w270:bool)
            n161 = case shown="False" w270 {
              tunnel: w272 -> [w273 w277]
              tunnel: [w273 w276] -> w271
              frame False {
                # "Don't bother trying to send a message to the RT system if UI Main VI isn't even connected"
              }
              frame True {
                n162 = global read "Global - UI Stream and Variable Connections.vi" "UI Command Stream"() -> (w274:refnum<k21>)
                n163 = shared-variable-write(w274, w277, T7 {"Message"="Update UI", "Message Data"=variant} ("data in")) -> (w276:errorcluster)  [unwired: 1 in, 2 out]
              }
            }
          }
          frame Enabled {
          }
        }
      }
      frame "Control" {
        # "Update various controls - Send control state/settings/setpoints to RT.\nNOTE: Add additional messages to this case for each new independeent control algorithm."
        n164 = disable-structure shown="Enabled" {
          disable-tunnel: w282 -> [w287 w295]
          disable-tunnel: w281 -> [w286 _]
          disable-tunnel: w280 -> [w285 _]
          disable-tunnel: [w283 w295] -> w279
          frame Disabled {
            n165 = local read "Connected?"() -> (w284:bool)
            n166 = case shown="True" w284 {
              tunnel: [w288 w289] -> w283
              tunnel: w287 -> [w288 w294]
              tunnel: w286 -> [_ w293]
              tunnel: w285 -> [_ w290]
              frame False {
              }
              frame True {
                n167 = global read "Global - UI Stream and Variable Connections.vi" "UI Command Stream"() -> (w292:refnum<k21>)
                n168 = Bundle(w293, "Message Data"=w290) -> (w291:cluster{string, "Message Data":variant})  [unwired: 1 in]
                n169 = shared-variable-write(w292, w294, w291) -> (w289:errorcluster)  [unwired: 1 in, 2 out]
              }
            }
          }
          frame Enabled {
          }
        }
      }
      frame "Critical Error", "Log-Only Error", "Non-Critical Error", "RT Error" {
        # "Error - Display message in status indicator on panel.  If it's a critical error, shut down this VI with an 'Exit' message."
        n170 = case shown="\"RT Error\"" w297 {
          selector: w297 -> [_ w314]
          tunnel: ["UI Error" w314] -> w296
          frame Default {
          }
          frame "RT Error" {
          }
        }
        n171 = Variant To Data(error in=w311, type=errorcluster {"status"=FALSE, "code"=0, "source"=""} ("error constant"), Variant=w309) -> (data=w304:errorcluster, error out=w310:errorcluster)
        n172 = Unbundle By Name(w304) -> ("code"=w303:i32, "source"=w307:string)
        n173 = Format Date/Time String() -> (date/time string=w306:string)  [unwired: 3 in]
        n174 = Format Into String(format string="\n%s: %s %d - %s", w306, w296, w303, w307) -> (resulting string=w298:string)  [unwired: 2 in, 1 out]
        n175 = call "Enqueue Message.vi"("error in (no error)"=w310, "Message Data"=w298, "Message"="Update System Status", "Message Queue"=w301) -> ("error out"=w302:errorcluster, "dup Message Queue"=w300:refnum<queue>)  [unwired: 6 in]
        n176 = case shown="\"Critical Error\"" w297 {
          tunnel: w302 -> [w315 w319]
          tunnel: w300 -> [_ w317]
          tunnel: [w315 w318] -> w312
          frame Default {
          }
          frame "Critical Error" {
            n177 = call "Enqueue Message.vi"("error in (no error)"=w319, "Message"="Exit", "Message Queue"=w317) -> ("error out"=w318:errorcluster)  [unwired: 7 in, 1 out]
          }
        }
      }
      frame "Update System Status" {
        # "#CodeRecommended - The code below ensures that the System Status string value does not become too large.  It uses the same maximum size as the RT error log to determine whether or not to remove the last half of the log string. Change this logic if you wish to maintain more/less of the information in the System Status string."
        # "Update System Status - Add a new string to the beginning of the System Status string on the UI."
        n178 = Variant To Data(error in=w330, type="", Variant=w328) -> (data=w325:string, error out=w329:errorcluster)
        n179 = local read "System Status"() -> (w323:string)
        n180 = global read "Global - Configuration Options.vi" "Error Log Max Size (bytes)"() -> (w321:i64)
        n181 = String Length(string=w323) -> (length=w324:i32)
        n182 = Greater?(x=w324, y=w321) -> (0:w322:bool)
        n183 = case shown="True" w322 {
          tunnel: w323 -> [w331 w335]
          tunnel: w321 -> [_ w334]
          tunnel: [w331 w336] -> w320
          frame False {
          }
          frame True {
            n184 = Divide(x=w334, y=i64 2) -> (x/y=w333:dbl)
            n185 = String Subset(string=w335, length (rest)=w333) -> (substring=w336:string)  [unwired: 1 in]
          }
        }
        n186 = Concatenate Strings(w325, w320) -> (→"System Status":string)
      }
      frame "Exit" {
        w337 = FALSE ("Connected?")
        # "Flush the Writer Stream to ensure all pending messages are sent to RT Main VI"
        # "Close all connections"
        # "Stop Monitoring Loop"
        # "Stop Event Handling Loop"
        # "Release the UI Message queue reference"
        # "Stop UI Message Loop"
        # "Exit - Fire the User Event to stop the Event Handling Loop, and toggle the global variable to stop the Monitoring Loop.  This message alone causes all three loops to stop."
        n187 = global write "Global - All UI Loop Stop.vi" "All UI Loop Stop"(TRUE ("Stop Monitoring Loop")) -> ()
        n188 = call "Fire User Event - Stop.vi"("User Event - Stop"=w349) -> ("error out"=w348:errorcluster)  [unwired: 10 in]
        n189 = property on="Controller\nAddress" class="Str"("DisabledEnum"=T6."Enabled" ("Disabled")) -> ()  [unwired: 2 in, 2 out]
        n190 = Release Queue(queue=w346, error in (no error)=w350) -> (error out=w347:errorcluster)  [unwired: 1 in, 2 out]
        n191 = global read "Global - UI Stream and Variable Connections.vi" "UI Command Stream"() -> (w342:refnum<k21>)
        n192 = global read "Global - UI Stream and Variable Connections.vi" "RT Message Stream"() -> (w344:refnum<k21>)
        n193 = global read "Global - UI Stream and Variable Connections.vi" "Variable References"() -> (w343:T8)
        n194 = Flush Stream(11:w342) -> (3:w341:refnum<k21>)  [unwired: 3 in, 2 out]
        n195 = Destroy Stream Endpoint(11:w344) -> (0:w338:errorcluster)  [unwired: 1 in]
        n196 = call "Close Variable Connections.vi"("Variable References"=w343) -> ()  [unwired: 11 in]
        n197 = Destroy Stream Endpoint(11:w341) -> (0:w339:errorcluster)  [unwired: 1 in]
        n198 = local write "Connected?"(w337) -> ()
        n199 = local write "Record?"(w337) -> ()
        n200 = Merge Errors(w348, w347) -> (w351:errorcluster)
      }
      frame "Close Connections" {
        # "Flush the Writer Stream to ensure all pending messages are sent to RT Main VI"
        # "Close Connections\nCALLED BY THE RT ONLY"
        n201 = property on="Controller\nAddress" class="Str"("DisabledEnum"=T6."Enabled" ("Disabled")) -> ()  [unwired: 2 in, 2 out]
        n202 = global read "Global - UI Stream and Variable Connections.vi" "UI Command Stream"() -> (w356:refnum<k21>)
        n203 = global read "Global - UI Stream and Variable Connections.vi" "RT Message Stream"() -> (w358:refnum<k21>)
        n204 = global read "Global - UI Stream and Variable Connections.vi" "Variable References"() -> (w357:T8)
        n205 = local write "Connected?"(FALSE ("Connected?")) -> ()
        n206 = Flush Stream(11:w356) -> (3:w355:refnum<k21>)  [unwired: 3 in, 2 out]
        n207 = Destroy Stream Endpoint(11:w358) -> ()  [unwired: 1 in, 1 out]
        n208 = call "Close Variable Connections.vi"("Variable References"=w357) -> ()  [unwired: 11 in]
        n209 = Destroy Stream Endpoint(11:w355) -> ()  [unwired: 1 in, 1 out]
        n210 = Merge Errors(w359) -> (w360:errorcluster)
      }
      frame "---Copy This Frame---" {
        # "Duplicate this frame when creating new messages.  Change this comment in the duplicated frame to describe this message."
        n211 = Merge Errors(w362) -> (w361:errorcluster)
      }
      frame Default {
        # "'Default' case only runs if there is a message that isn't defined in any of the other cases.  Output a programming error."
        n212 = Format Into String(format string="The invalid message string \"%s\" was received in the Message Handling Loop." ("Invalid Message Loop Message"), w366) -> (resulting string=w363:string)  [unwired: 2 in, 1 out]
        n213 = call <vilib>:"Error Cluster From Error Code.vi"("error message (\"\")"=w363, "error code (0)"=1) -> ("error out"=w364:errorcluster)  [unwired: 7 in]
      }
    }
    n214 = Concatenate Strings(w155, "\r\n", w153) -> (w152:string)
    "message log" <- w152
    n215 = call "UI Error Handler - Message Handler.vi"("error in (no error)"=w157, "Message Queue"=w158) -> ()  [unwired: 9 in, 1 out]
    n216 = call <vilib>:"Clear Errors.vi"("error in (no error)"=w157) -> ("error out"=w156:errorcluster)  [unwired: 5 in, 1 out]
    n217 = Wait Until Next ms Multiple(millisecond multiple=u32 50) -> ()  [unwired: 1 out]
  }
  n218 = while {
    tunnel: w1 -> [w368]
    tunnel: [w371] -> w14
    shift-right: [w369] -> w6
    shift-left: w12 -> [w370]
    stop <- w372 stop-if-true
    # "Event Handling Loop"
    n219 = event shown="[14] \"Temp Alert\": Value Change" {
      selector: w370 -> [_ _ _ _ _ _ _ _ _ _ _ _ _ _ _ _]
      dyn-events: [_ _ _ _ _ _ _ _ _ _ _ _ _ _ _ _] -> w369
      timeout: _ -> [_ _ _ _ _ _ _ _ _ _ _ _ _ _ _ _]
      tunnel: [_ _ TRUE ("Discard?") _ _ _ _ _ _ _ _ _ _ _ _ _] -> w373
      tunnel: w368 -> [w380 w382 _ _ _ _ _ _ _ _ _ _ _ _ _ _]
      tunnel: [w381 w385 _ w387 w390 w392 w393 w395 w398 w399 w402 w406 w409 w410 w412 w414] -> w371
      event "Connect to Controller": Value Change {
        n220 = event-data() -> ()  [unwired: 1 in, 1 out]
        n221 = call "Enqueue Message.vi"("Message"="Connect", "Message Queue"=w380) -> ("error out"=w381:errorcluster)  [unwired: 8 in, 1 out]
      }
      event "Exit": Value Change {
        w383 = TRUE  # Priority Message
        # "The UI Message Loop handles sending the Exit message to other loops."
        n222 = event-data() -> ()  [unwired: 1 in, 1 out]
        n223 = call "Enqueue Message.vi"("Priority Message? (F)"=w383, "Message"="Exit", "Message Queue"=w382) -> ("error out"=w385:errorcluster)  [unwired: 7 in, 1 out]
      }
      event User Event {
        # "The Message Handling Loop processed an \"Exit\" message, which fired this event to stop the Event Handling Loop."
        n224 = event-data() -> ()  [unwired: 1 in, 1 out]
      }
      event "Pump Frequency Cmd [Hz]": Value Change {
        n225 = event-data() -> ()  [unwired: 1 in, 1 out]
        n226 = shared-variable "NI-cRIO-9035-01C89D95\\Mod5\\Pump Frequency Cmd [Hz]"("Pump Frequency Cmd [Hz]") -> (error out=w387:errorcluster)  [unwired: 1 in]
      }
      event "Drive Air Pressure Cmd [psig]": Value Change {
        n227 = event-data() -> ()  [unwired: 1 in, 1 out]
        n228 = shared-variable "NI-cRIO-9035-01C89D95\\Mod5\\Drive Air Pressure Cmd"("Drive Air Pressure Cmd [psig]") -> (error out=w390:errorcluster)  [unwired: 1 in]
      }
      event "Recirc Valve % Closed Cmd": Value Change {
        n229 = event-data() -> ()  [unwired: 1 in, 1 out]
        n230 = shared-variable "NI-cRIO-9035-01C89D95\\Mod5\\Recirc Valve % Closed Cmd"("Recirc Valve % Closed Cmd") -> (error out=w392:errorcluster)  [unwired: 1 in]
      }
      event "Flow Valve % Closed Cmd": Value Change {
        n231 = event-data() -> ()  [unwired: 1 in, 1 out]
        n232 = shared-variable "NI-cRIO-9035-01C89D95\\Mod5\\Flow Valve % Closed Cmd"("Flow Valve % Closed Cmd") -> (error out=w393:errorcluster)  [unwired: 1 in]
      }
      event "Cooling Valve % Closed Cmd": Value Change {
        n233 = event-data() -> ()  [unwired: 1 in, 1 out]
        n234 = shared-variable "NI-cRIO-9035-01C89D95\\Mod5\\Recup Bypass Valve % Closed Cmd"("Cooling Valve % Closed Cmd") -> (error out=w395:errorcluster)  [unwired: 1 in]
      }
      event "Drive Air Enable": Value Change {
        n235 = event-data() -> ()  [unwired: 1 in, 1 out]
        n236 = shared-variable "NI-cRIO-9035-01C89D95\\Mod1\\Drive Air Enable"("Drive Air Enable") -> (error out=w398:errorcluster)  [unwired: 1 in]
      }
      event "Pump Enable": Value Change {
        n237 = event-data() -> ()  [unwired: 1 in, 1 out]
        n238 = shared-variable "NI-cRIO-9035-01C89D95\\Mod1\\Pump Enable"("Pump Enable") -> (error out=w399:errorcluster)  [unwired: 1 in]
      }
      event "Vent Valve": Value Change {
        n239 = event-data() -> ()  [unwired: 1 in, 1 out]
        n240 = Not(x="Vent Valve") -> (.not. x?=w404:bool)
        n241 = shared-variable "NI-cRIO-9035-01C89D95\\Mod1\\Close Vent Valve"(w404) -> (error out=w401:errorcluster)  [unwired: 1 in]
        n242 = shared-variable "NI-cRIO-9035-01C89D95\\Mod1\\Open Vent Valve"("Vent Valve") -> (error out=w405:errorcluster)  [unwired: 1 in]
        n243 = Merge Errors(w401, w405) -> (w402:errorcluster)
      }
      event "Heater Power Cmd [%]": Value Change {
        n244 = event-data() -> ()  [unwired: 1 in, 1 out]
        n245 = shared-variable "NI-cRIO-9035-01C89D95\\Mod5\\Heater Power Cmd [%]"("Heater Power Cmd [%]") -> (error out=w406:errorcluster)  [unwired: 1 in]
      }
      event "Regulated CO2 Pressure Cmd [psig]": Value Change {
        n246 = event-data() -> ()  [unwired: 1 in, 1 out]
        n247 = shared-variable "NI-cRIO-9035-01C89D95\\Mod5\\Supply CO2 Pressure Cmd"("Regulated CO2 Pressure Cmd [psig]") -> (error out=w409:errorcluster)  [unwired: 1 in]
      }
      event "Water Valve % Closed Cmd": Value Change {
        n248 = event-data() -> ()  [unwired: 1 in, 1 out]
        n249 = shared-variable "NI-cRIO-9035-01C89D95\\Mod5\\Water Valve % Closed Cmd"("Water Valve % Closed Cmd") -> (error out=w410:errorcluster)  [unwired: 1 in]
      }
      event "Temp Alert": Value Change {
        n250 = event-data() -> ()  [unwired: 1 in, 1 out]
        n251 = shared-variable "NI-cRIO-9035-01C89D95\\Mod1\\Temperature Alert"("Temp Alert") -> (error out=w412:errorcluster)  [unwired: 1 in]
      }
      event "Alarm": Value Change {
        n252 = event-data() -> ()  [unwired: 1 in, 1 out]
        n253 = shared-variable "NI-cRIO-9035-01C89D95\\Mod1\\Status Alarm"("Alarm") -> (error out=w414:errorcluster)  [unwired: 1 in]
      }
    }
    n254 = case shown="Error" w371 {
      tunnel: [w374 TRUE ("Discard?")] -> w372
      tunnel: w373 -> [w374 _]
      tunnel: w368 -> [_ w375]
      frame No Error {
      }
      frame Error {
        # "On error, send Exit message, and stop loop."
        n255 = call "Enqueue Message.vi"("Priority Message? (F)"=TRUE ("Discard?"), "Message"="Exit", "Message Queue"=w375) -> ()  [unwired: 7 in, 2 out]
      }
    }
  }
  n256 = Unregister For Events(event registration refnum=w6, error in=w14) -> (error out=w7:errorcluster)
  n257 = Merge Errors(w7, w15) -> (w13:errorcluster)
  n258 = call "Destroy User Event - Stop.vi"("error in (no error)"=w13, "User Event - Stop"=w11) -> ("error out"=w5:errorcluster)  [unwired: 9 in]
  n259 = call <vilib>:"Simple Error Handler.vi"("error in (no error)"=w5) -> ("error out"=w3:errorcluster)  [unwired: 4 in, 4 out]
  n260 = disable-structure shown="Default" {
    disable-tunnel: w3 -> [_ _]
    frame condition #0 {
      # "Call Quit LabVIEW if running as a built application."
      n261 = Quit LabVIEW() -> ()  [unwired: 1 in]
    }
    frame condition #1 (active) {
      n262 = local write "Connect to Controller"(FALSE ("Connect to Controller")) -> ()
    }
  }
